vi "Super Talon Test 2016.vi"() -> ()   [LabVIEW 2015]
doc: "This example shows how to control motor speed using CAN Jaguar and a quadrature encoder. For details setting up and understanding CAN Jaguar, see the Can Jaguar Fundamentals tutorial accessable from the LabVIEW Getting Started Window.\n\nTo control the motor speed, a PID control loop runs on the Jaguar. Notice that the encoder is wired directly to the Jaguar. One advantage of this is that the PID control does not use resources on the roboRIO. One disadvantage is that the PID code cannot be viewed or changed. However, the control can be tuned by changing the PID Parameters.\n\nOn the diagram, notice that the PID tuning parameters are only applied once before the motor is enabled. To learn about changing PID parameters while the program is running, see the CAN Position Control Encoder example. Since the control loop runs on the Jaguar, the LabVIEW loop delay is set to a slow 100ms. In fact the only reason this loop needs to run is to send a new set speed and read the actual speed.\n\nCorrect tuning parameters for a PID controller are dependent on the complete system of the motor and the load. It will be difficult to tune this system if there is no load attached to the motor. While this example is not a PID tutorial, the following information may help in understanding how to tune your PID control system.\n\nP (proportional) depends on the present error, I (integral) on the accumulation of past errors, and D (derivative) is a prediction of future errors, based on the current rate of change. The proportional parameter (P) will reduce the rise time and will reduce, but never eliminate, the steady-state error. The integral parameter (I) will eliminate the steady-state error, but may make the transient response worse. The derivative parameter (D) will increase the stability of the system, reducing the overshoot, and improving the transient response. The effects of each parameter are summarized in a table on the front panel.\n\nThis example expects a USB cable connected from your development PC to the Type B USB Jack (next to the power input) on the roboRIO.\n\nThis example requires the Driver Station to be running with Teleoperated Enabled."
uses:
  <vilib>/Rock Robotics/WPI/CAN/TalonSRX/WPI_CANTalonSRX_APIControlMode.ctl
  <vilib>/Rock Robotics/WPI/CAN/TalonSRX/WPI_CANTalonSRX_APIFeedbackSelect.ctl
  <vilib>/Rock Robotics/WPI/MotorControl/WPI_MotorControlOpenCANTalonSRX.vi
panel:
  in  "Stop All":bool
  in  "Start All":bool
  in  "Tab Control 2":T1(tab)
  out "Actual Speed (RPM)":dbl
  in  "P":dbl=1.0
  in  "D":dbl
  in  "F":dbl=0.01
  in  "I":dbl
  in  "Target Value":dbl
  out "Actual Position (Rotations)":dbl
  out "Percent VBus":dbl
  out "A/D Value":dbl
  out "Test Running":string
  in  "Control Mode":string(combo)
  in  "Motor Address":u64
  in  "Tab Control":T2(tab)
  out "Voltage Feedback Chart":cluster{dbl, dbl}(graph)
  out "Speed Feedback Chart":cluster{dbl, dbl}(graph)
  out "Position Feedback Chart":cluster{dbl, dbl}(graph)
  out "Potentiometer Position Feedback":cluster{dbl, dbl}(graph)
  in  "Stop Motor 1":bool
  in  "Forward Limit Switch":bool
  in  "Reverse Limit Switch":bool
  in  "Switches Normally Open":bool
  in  "Start Motor 1":bool
  in  "I Zone":dbl=0.01
  in  "I Zone 2":dbl=0.01
  in  "Start Motor 2":bool
  in  "Motor Address 2":u64
  in  "Control Mode 2":string(combo)
  in  "Target Value 2":dbl
  in  "I 2":dbl
  in  "F 2":dbl=0.01
  in  "D 2":dbl caption="D"
  in  "P 2":dbl=1.0 caption="P"
  out "Test Running 2":string
  out "Percent VBus 2":dbl
  out "A/D Value 2":dbl
  out "Actual Speed (RPM) 2":dbl
  out "Actual Position (Rotations) 2":dbl
  in  "Switches Normally Open 2":bool
  in  "Reverse Limit Switch 2":bool
  in  "Forward Limit Switch 2":bool
  in  "Tab Control 3":T2(tab)
  out "Voltage Feedback Chart 2":cluster{dbl, dbl}(graph)
  out "Speed Feedback Chart 2":cluster{dbl, dbl}(graph)
  out "Position Feedback Chart 2":cluster{dbl, dbl}(graph)
  out "Potentiometer Position Feedback 2":cluster{dbl, dbl}(graph)
  in  "Stop Motor 2":bool
  in  "I Zone 3":dbl=0.01
  in  "Start Motor 3":bool
  in  "Motor Address 3":u64
  in  "Control Mode 3":string(combo)
  in  "Target Value 3":dbl
  in  "I 3":dbl
  in  "F 3":dbl=0.01
  in  "D 3":dbl caption="D"
  in  "P 3":dbl=1.0 caption="P"
  out "Test Running 3":string
  out "Percent VBus 3":dbl
  out "A/D Value 3":dbl
  out "Actual Speed (RPM) 3":dbl
  out "Actual Position (Rotations) 3":dbl
  in  "Switches Normally Open 3":bool
  in  "Reverse Limit Switch 3":bool
  in  "Forward Limit Switch 3":bool
  in  "Tab Control 4":T2(tab)
  out "Voltage Feedback Chart 3":cluster{dbl, dbl}(graph)
  out "Speed Feedback Chart 3":cluster{dbl, dbl}(graph)
  out "Position Feedback Chart 3":cluster{dbl, dbl}(graph)
  out "Potentiometer Position Feedback 3":cluster{dbl, dbl}(graph)
  in  "Stop Motor 3":bool
  in  "I Zone 4":dbl=0.01
  in  "Start Motor 4":bool
  in  "Motor Address 4":u64
  in  "Control Mode 4":string(combo)
  in  "Target Value 4":dbl
  in  "I 4":dbl
  in  "F 4":dbl=0.01
  in  "D 4":dbl caption="D"
  in  "P 4":dbl=1.0 caption="P"
  out "Test Running 4":string
  out "Percent VBus 4":dbl
  out "A/D Value 4":dbl
  out "Actual Speed (RPM) 4":dbl
  out "Actual Position (Rotations) 4":dbl
  in  "Switches Normally Open 4":bool
  in  "Reverse Limit Switch 4":bool
  in  "Forward Limit Switch 4":bool
  in  "Stop Motor 4":bool
  in  "Tab Control 5":T2(tab)
  out "Voltage Feedback Chart 4":cluster{dbl, dbl}(graph)
  out "Speed Feedback Chart 4":cluster{dbl, dbl}(graph)
  out "Position Feedback Chart 4":cluster{dbl, dbl}(graph)
  out "Potentiometer Position Feedback 4":cluster{dbl, dbl}(graph)
  out "Error Out":errorcluster
  in  "Error In":errorcluster
  # "Set these inputs before running."
  # "Tuning parameters"
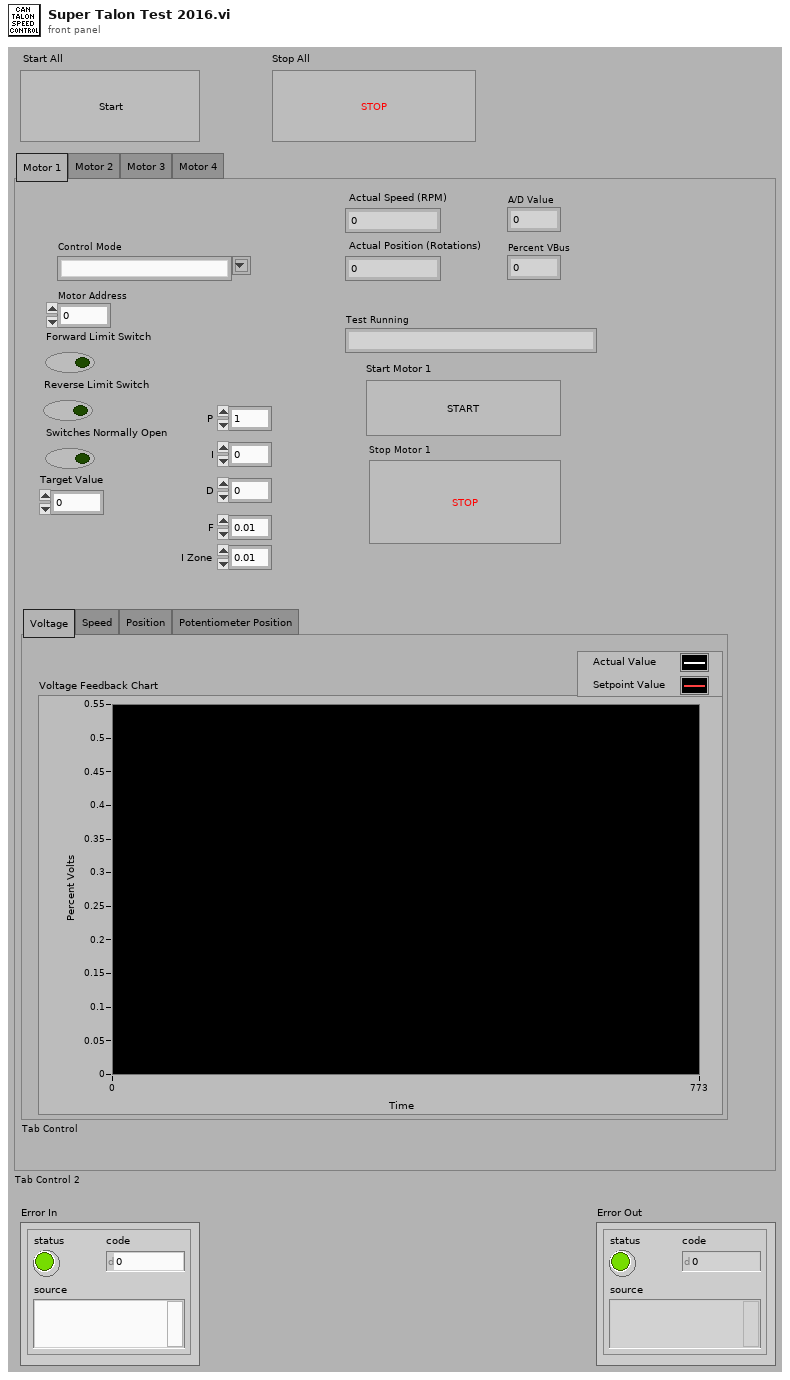
[diagram p1: front panel]
types:
  T1 = enum32{"Motor 1", "Motor 2", "Motor 3", "Motor 4"}
  T2 = enum32{"Voltage", "Speed", "Position", "Potentiometer Position"}
  T3 = typedef "WPI_CANTalonSRX_APIFeedbackSelect.ctl" = enum16{"Digital Quadrature Encoder", "Analog Potentiometer", "Analog Encoder", "Count on Quad-A (Rising-Edge)", "Count on Quad-A (Falling-Edge)", "CTR Magnetic Enc (Absolute)", "CTR Magnetic Enc (Relative)", "Pulse Width"}
  T4 = typedef "WPI_CANTalonSRX_APIControlMode.ctl" = enum8{"Percent VBus", "Speed", "Position", "Slave", "Unchanged / Invalid", "Voltage Compensation", "Current", "Motion Profile"}
  T5 = typedef "WPI_MotorControlDeviceRef.ctl" = cluster{"DeviceStatus":errorcluster, "Type":T6, "PWM":cluster{"PWM Channel":T7, "DeadBand":T8}, "CAN":cluster{"Device Number":u8, "Control Mode":T9, "Semaphore":T10, "Max Vout":dbl, "TalonSRX Control Mode":T4}, "Invert":bool}
  T6 = typedef "WPI_MotorControlType.ctl" = enum16{"PWM", "CAN", "CANTalonSRX"}
  T7 = typedef "FPGA_DIOPWMChannel.ctl" = enum8{"PWM 0", "PWM 1", "PWM 2", "PWM 3", "PWM 4", "PWM 5", "PWM 6", "PWM 7", "PWM 8", "PWM 9", "PWM MXP 0", "PWM MXP 1", "PWM MXP 2", "PWM MXP 3", "PWM MXP 4", "PWM MXP 5", "PWM MXP 6", "PWM MXP 7", "PWM MXP 8", "PWM MXP 9", "Invalid"}
  T8 = typedef "WPI_PWMDeadband.ctl" = cluster{"Name":string, "maxPositivePwm":i32, "minPositivePwm":i32, "centerPwm":i32, "maxNegativePwm":i32, "minNegativePwm":i32, "angularRange":u16}
  T9 = typedef "WPI_CANJaguar_ControlMode.ctl" = enum8{"Percent VBus", "Current", "Speed", "Position", "Voltage"}
  T10 = typedef "Semaphore RefNum" = refnum<k1>
  T11 = typedef "WPI_CANTalonSRX_GlobalStatus.ctl" = cluster{"Applied Throttle":dbl, "Module Enabled":bool, "CAN Error":errorcluster, "Closed Loop Error":dbl, "Forward Limit Switch Closed":bool, "Reverse Limit Switch Closed":bool, "Sensor Position":dbl, "Sensor Velocity":dbl, "Current":dbl, "Sticky Fault - Over Temp":bool, "Sticky Fault - Under Voltage":bool, "Sticky Fault - Forward Limit":bool, "Sticky Fault - Reverse Limit":bool, "Sticky Fault - Forward Soft Limit":bool, "Sticky Fault - Reverse Soft Limit":bool, "Brake is Enabled":bool, "Encoder Position":dbl, "Encoder Velocity":dbl, "Encoder Index Count":dbl, "Encoder A Pin State":bool, "Encoder B Pin State":bool, "Encoder Index Pin State":bool, "Analog In":dbl, "Analog In Velocity":dbl, "Temperature (C)":dbl, "Battery Voltage":dbl, "Control 5 Is Supported":bool, "Current Profile Slot Select":dbl, "Pos Div 8":bool, "Vel Div 4":bool, "Pulse Width Position":i32, "Pulse Width Velocity":i32, "Pulse Width Rise To Rise (us)":i32, "Pulse Width Rise To Fall (us)":i32, "Mot Prof Active Is Under Run":bool, "Mot Prof Active Has Under Run":bool, "Mot Prof Active Is Last":bool, "Mot Prof Active Velocity Only":bool, "Mot Prof Active Is Valid":bool, "Mot Prof Buffer Is Full":bool, "Mot Prof Active Profile Slot Select":i32, "Mot Prof NextID":i32, "Mot Prof Count":i32, "Mot Prof Active Velocity":dbl, "Mot Prof Active Position":dbl, "Mot Prof Output Enable":i32}
  T12 = cluster{"Applied Throttle":dbl, "Target Value 2":dbl}
  T13 = cluster{"Applied Throttle":dbl, "Target Value":dbl}
  T14 = cluster{"Applied Throttle":dbl, "Target Value 3":dbl}
  T15 = cluster{"Applied Throttle":dbl, "Target Value 4":dbl}
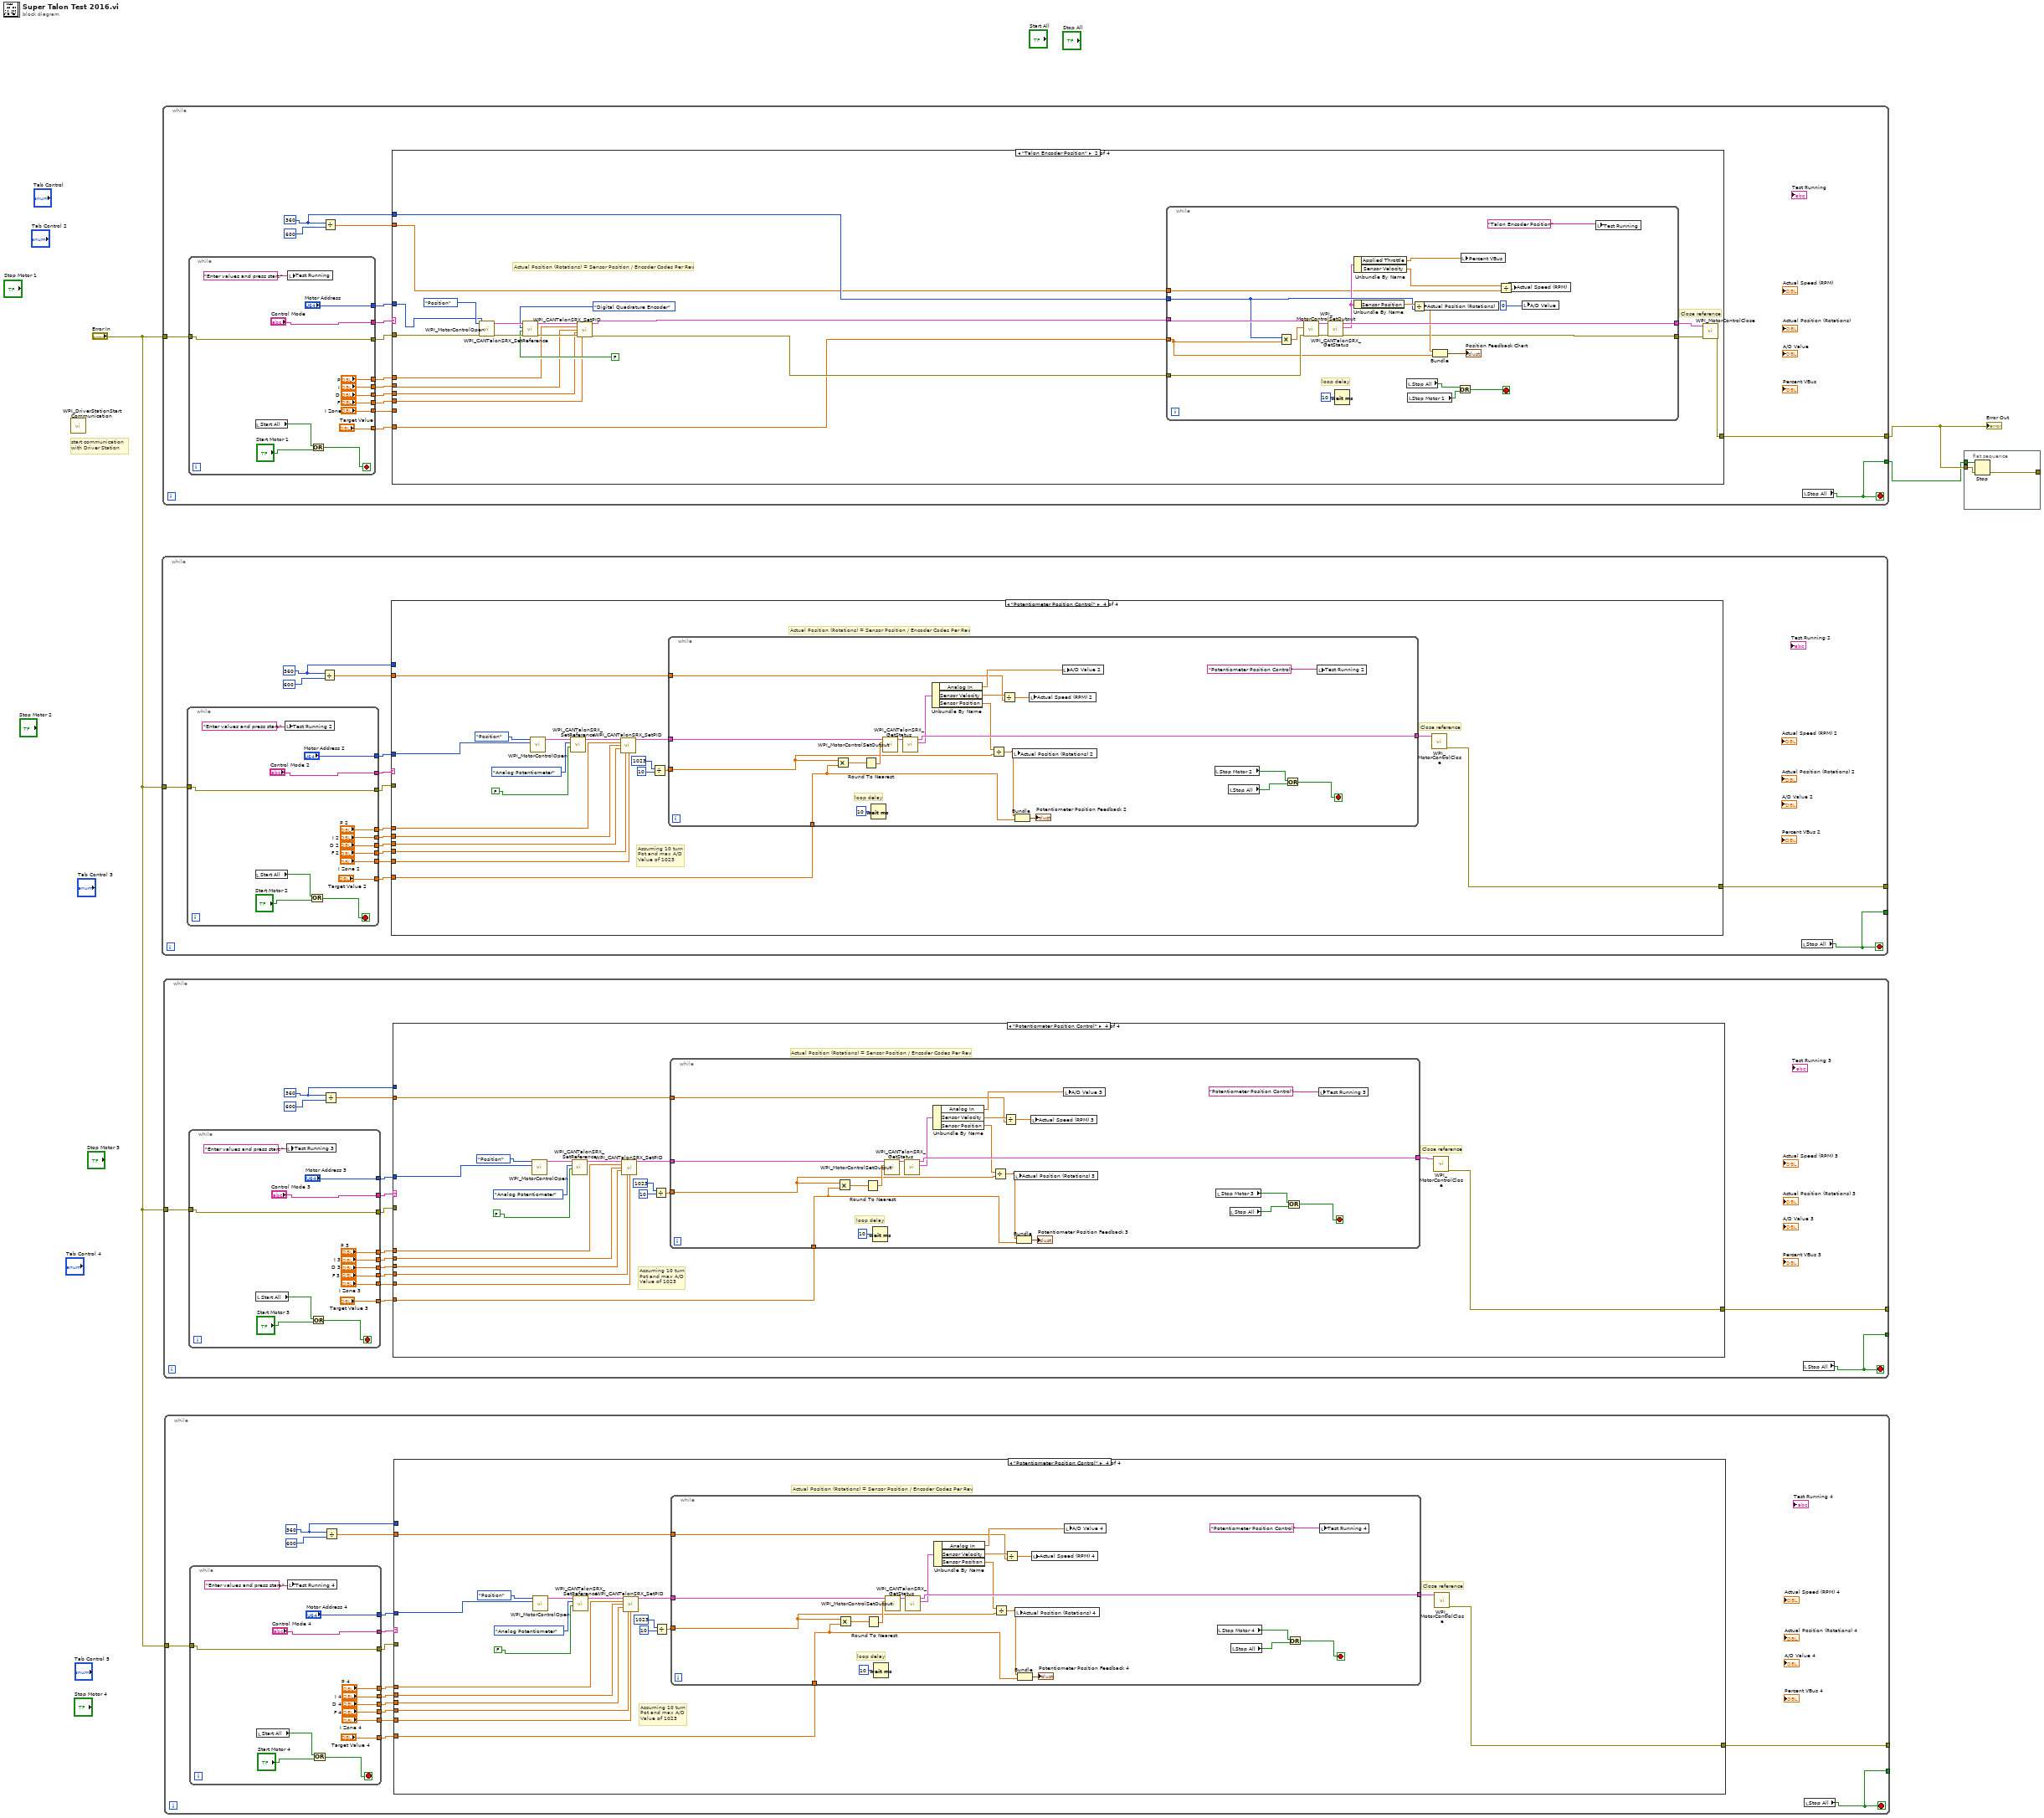
[diagram p0: block diagram]
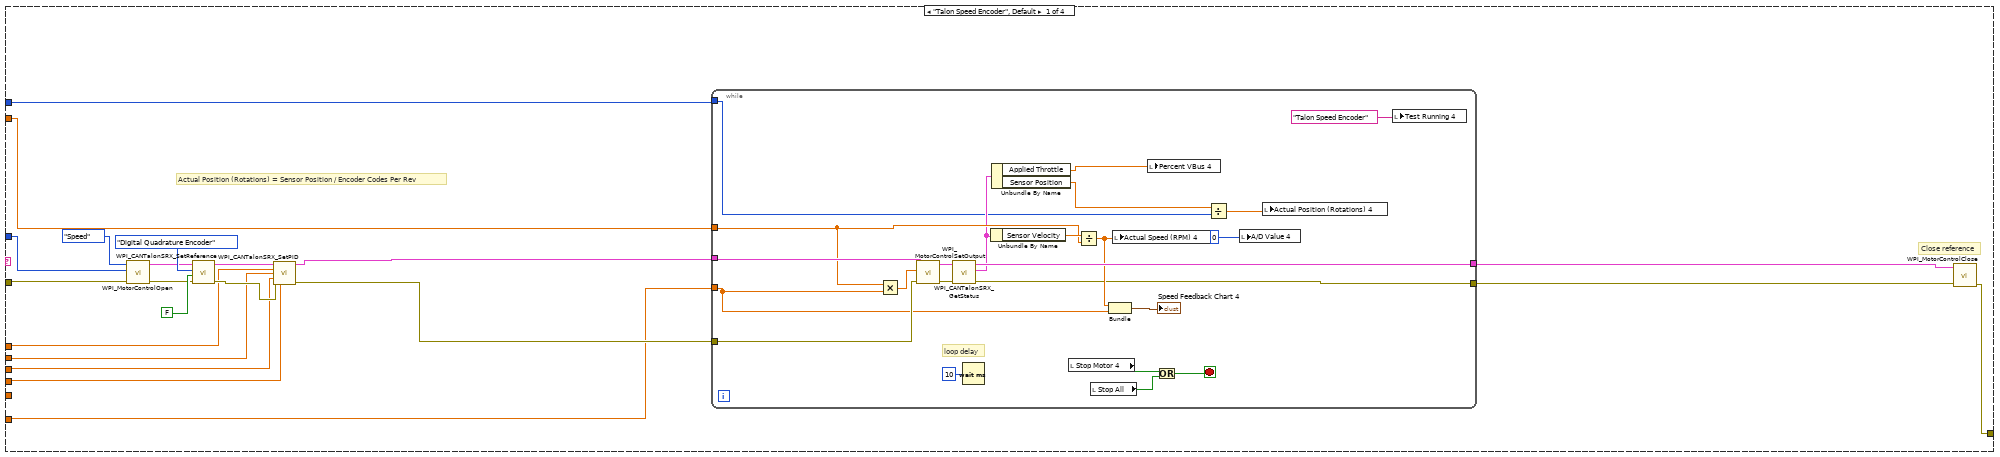
[diagram p2: hidden frame]
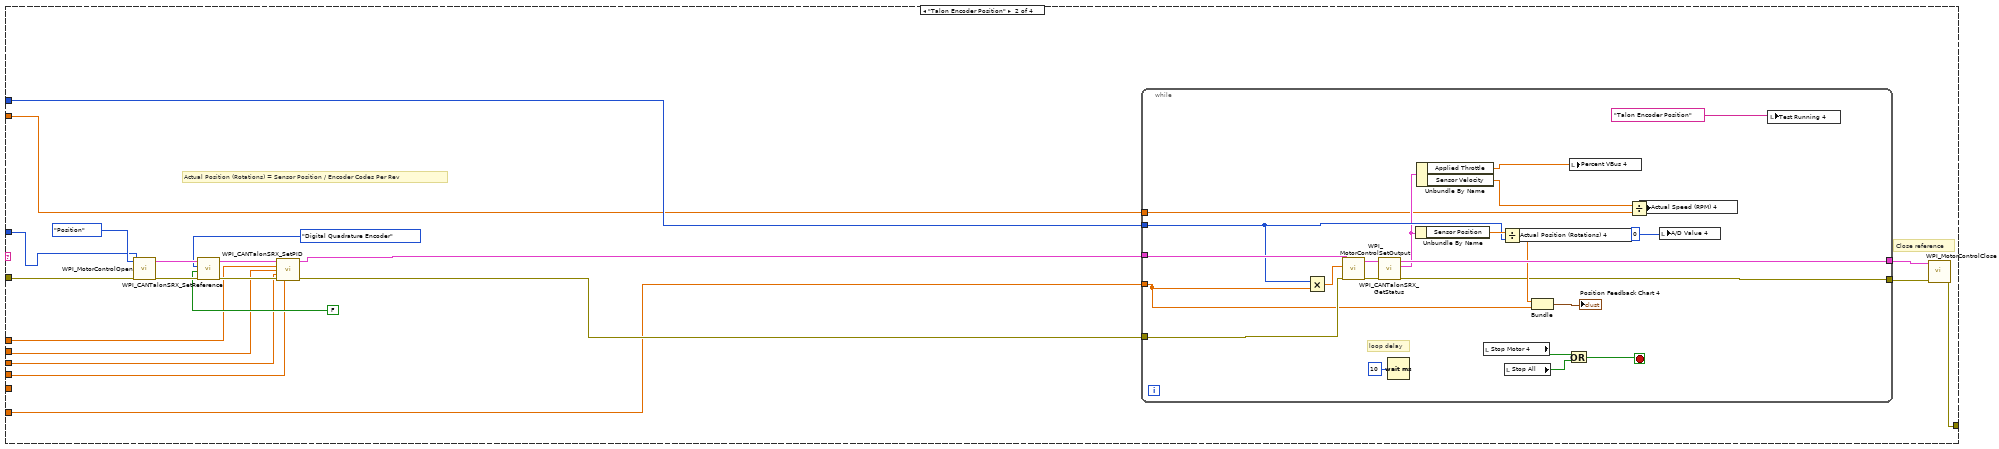
[diagram p3: hidden frame]
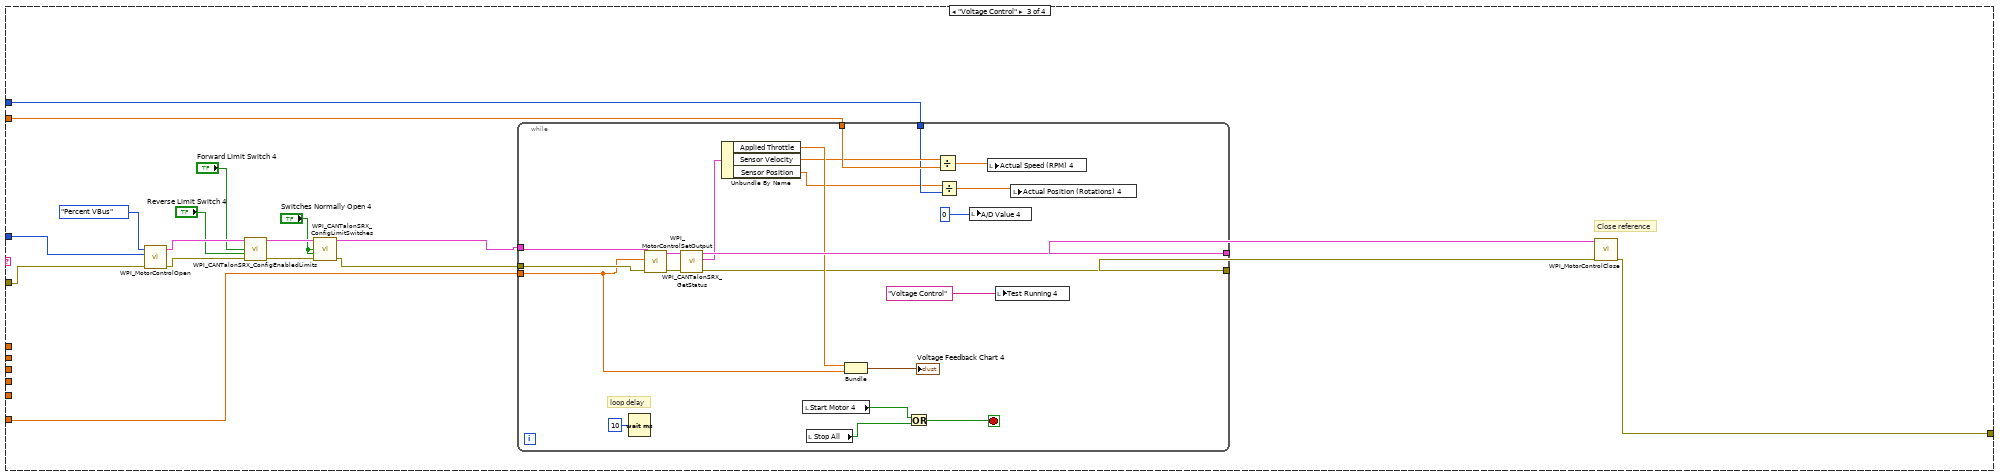
[diagram p4: hidden frame]
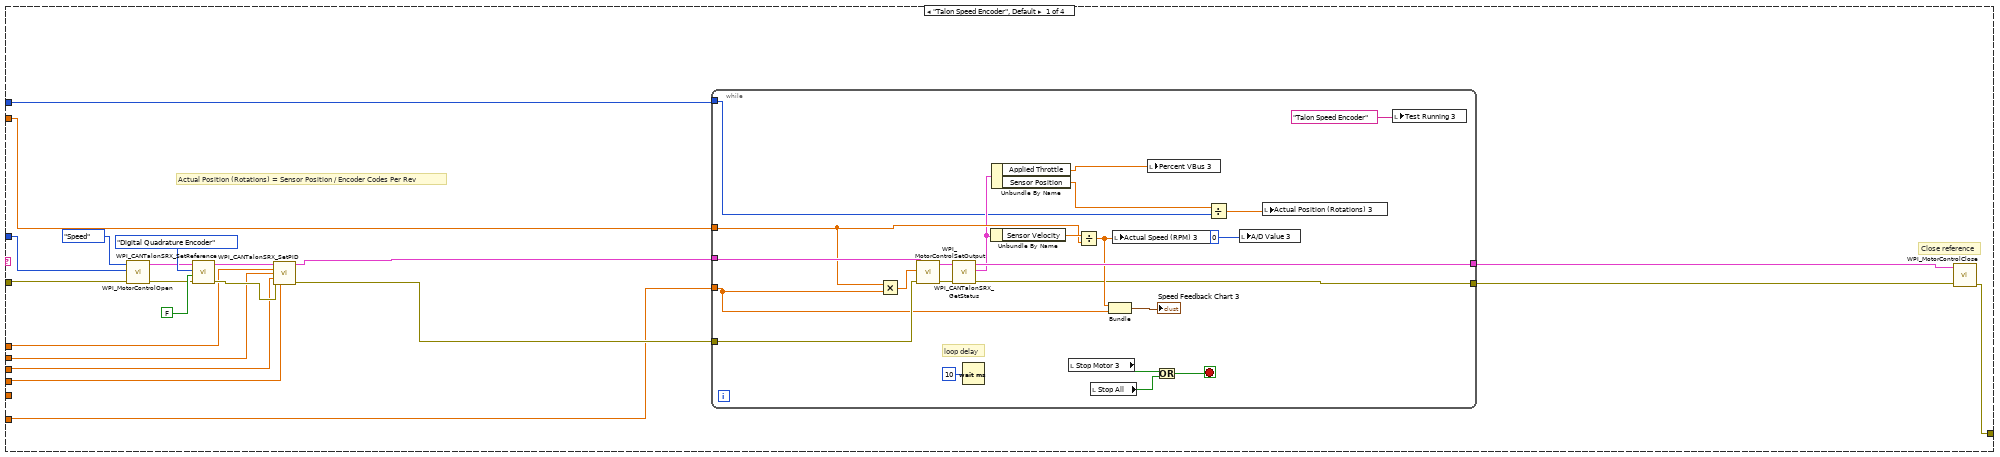
[diagram p5: hidden frame]
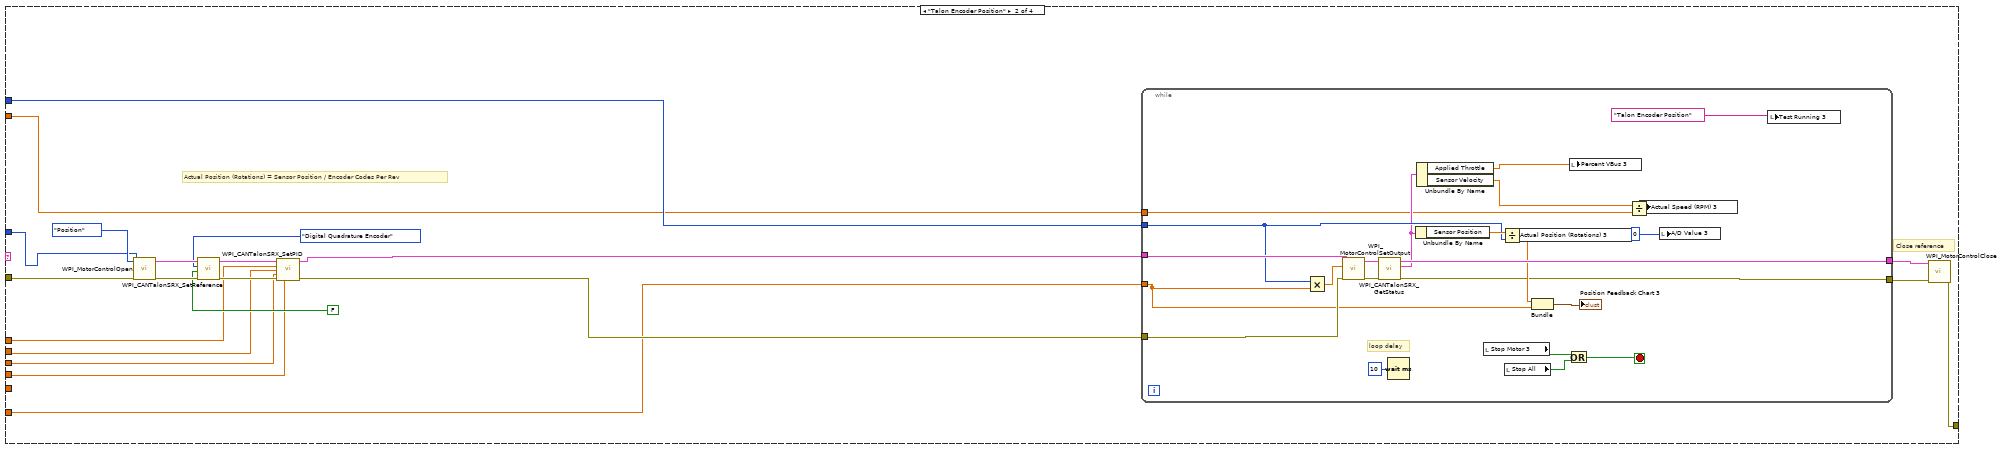
[diagram p6: hidden frame]
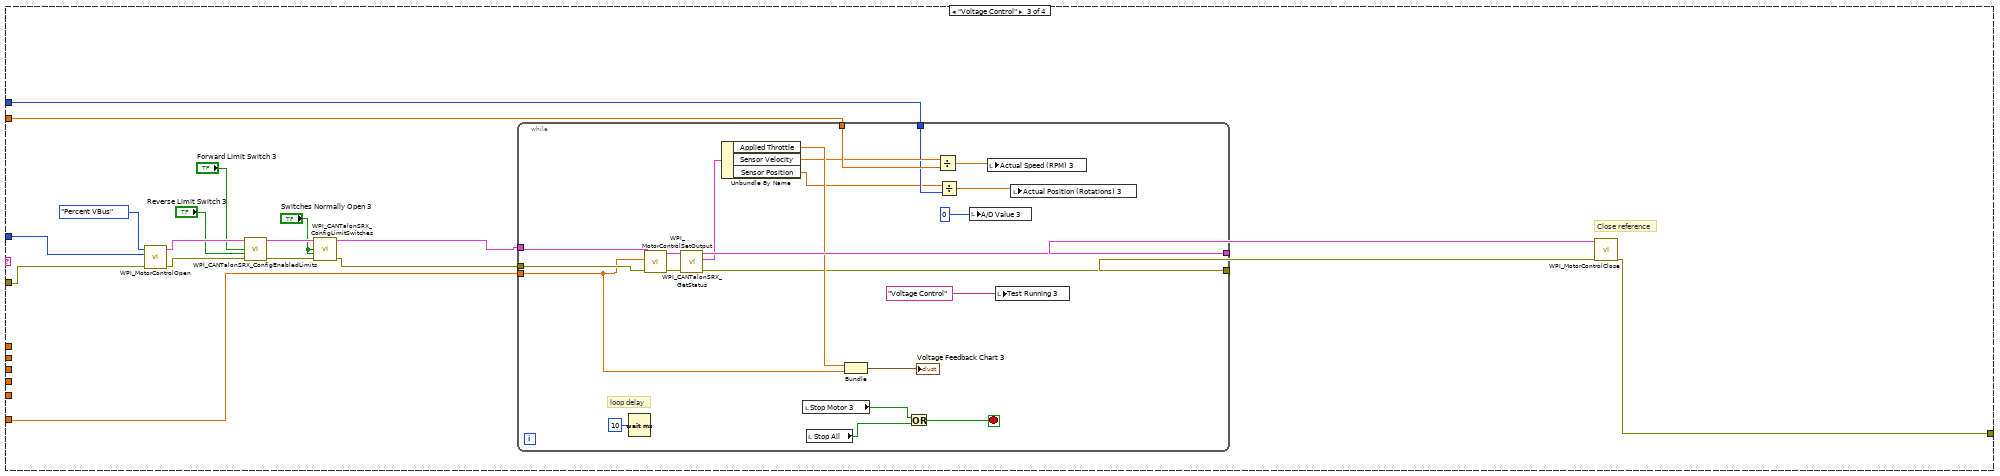
[diagram p7: hidden frame]
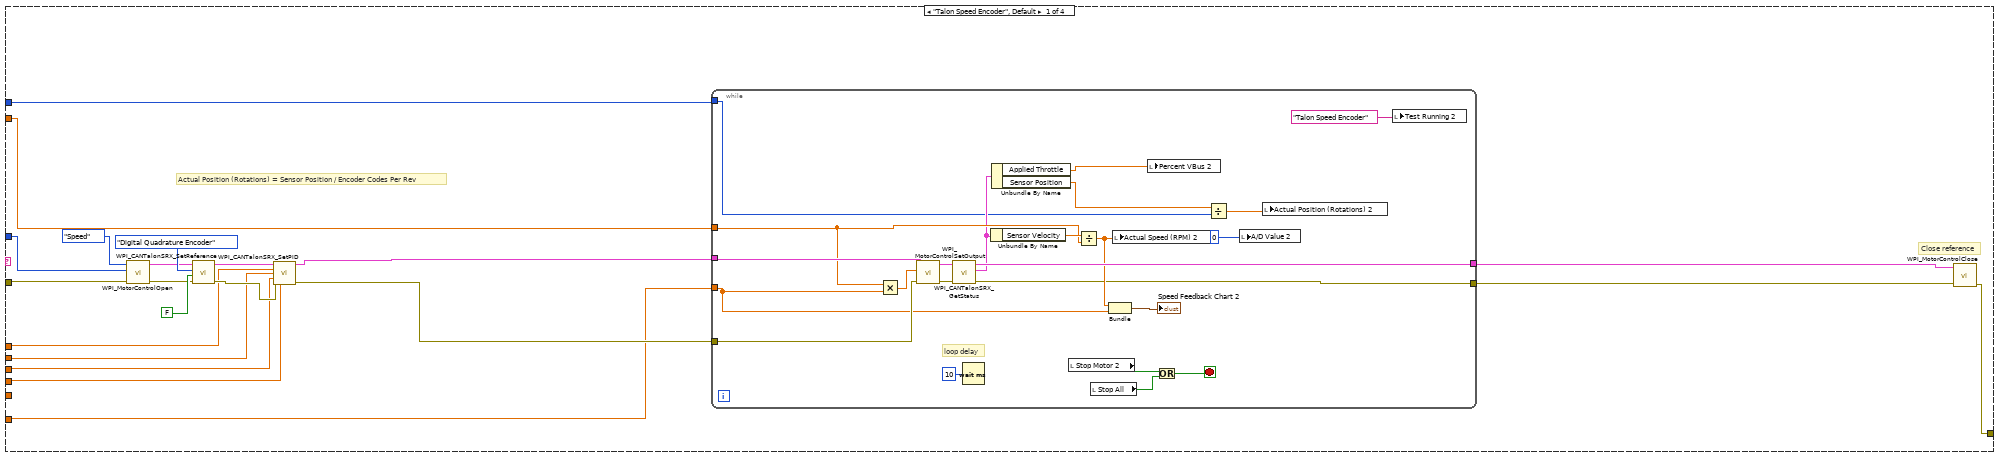
[diagram p8: hidden frame]
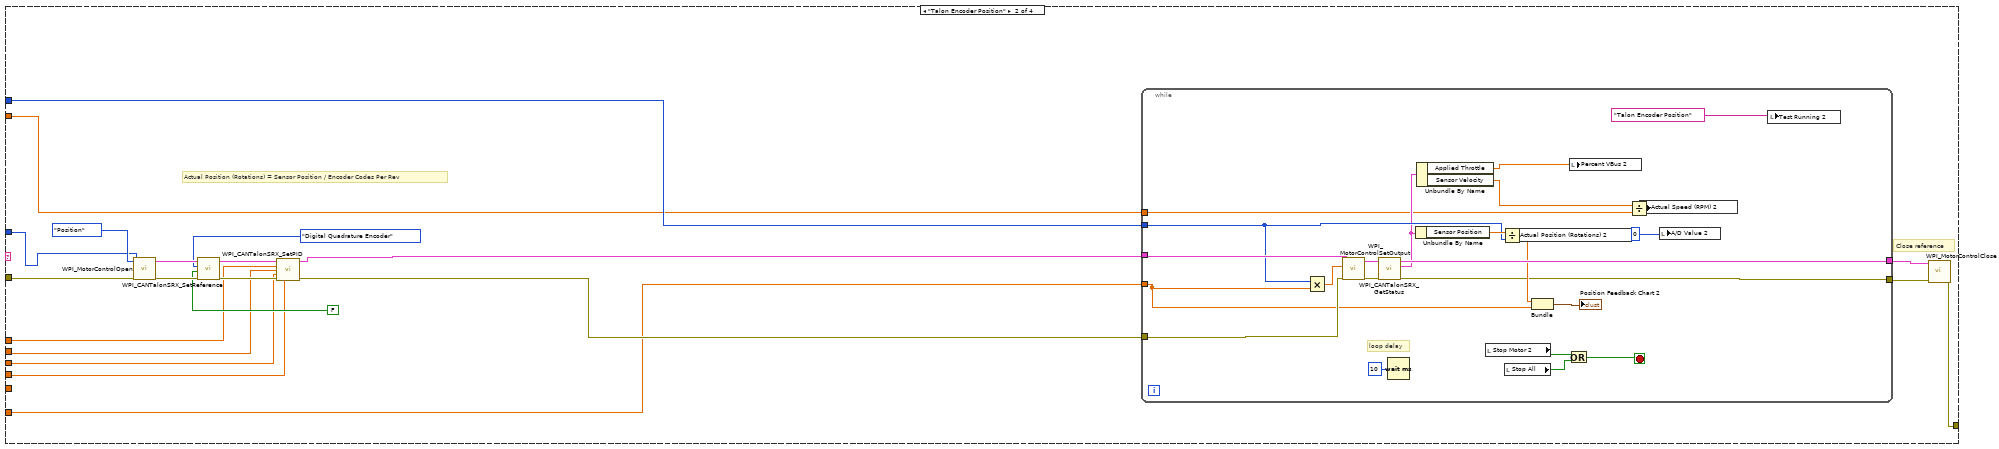
[diagram p9: hidden frame]
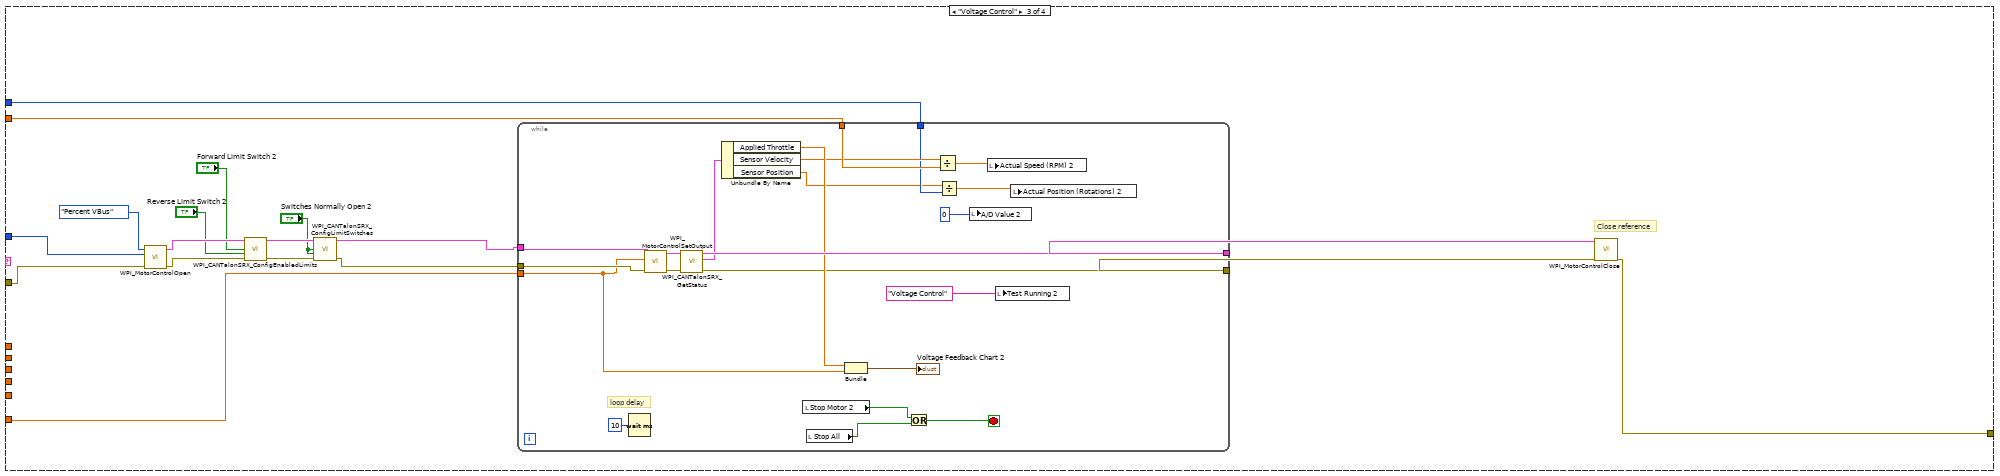
[diagram p10: hidden frame]
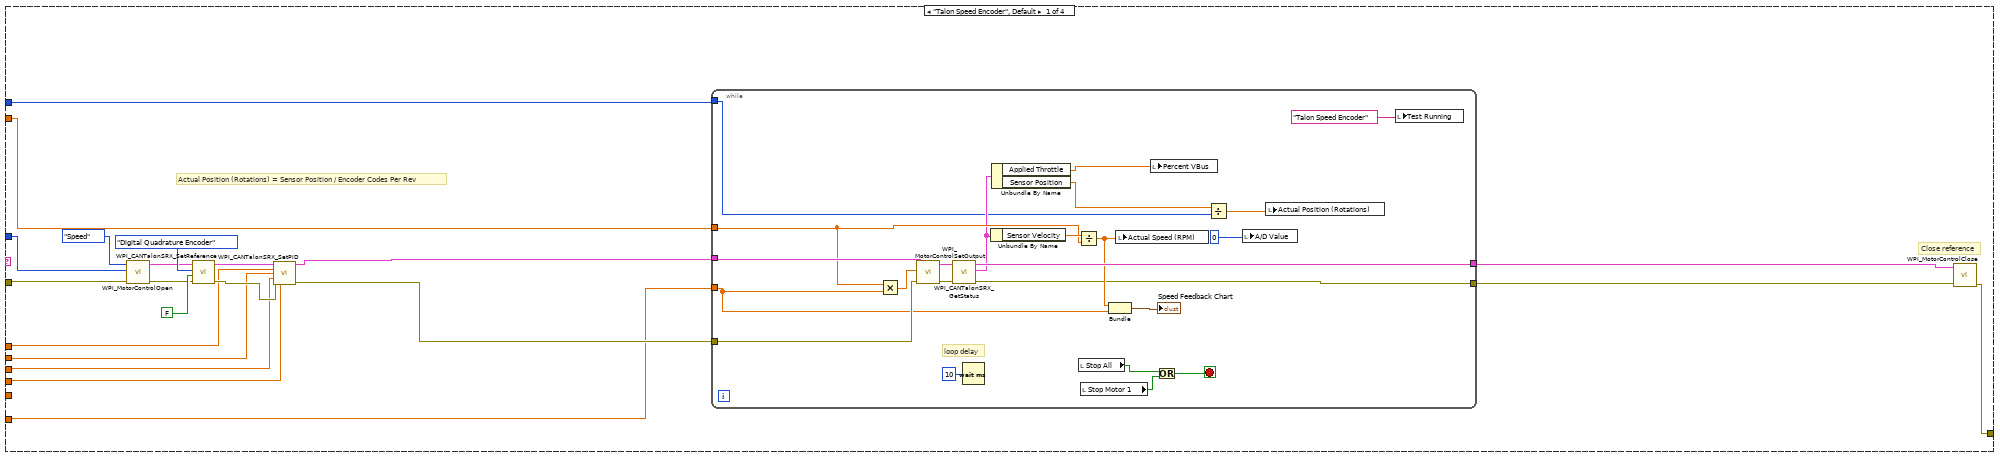
[diagram p11: hidden frame]
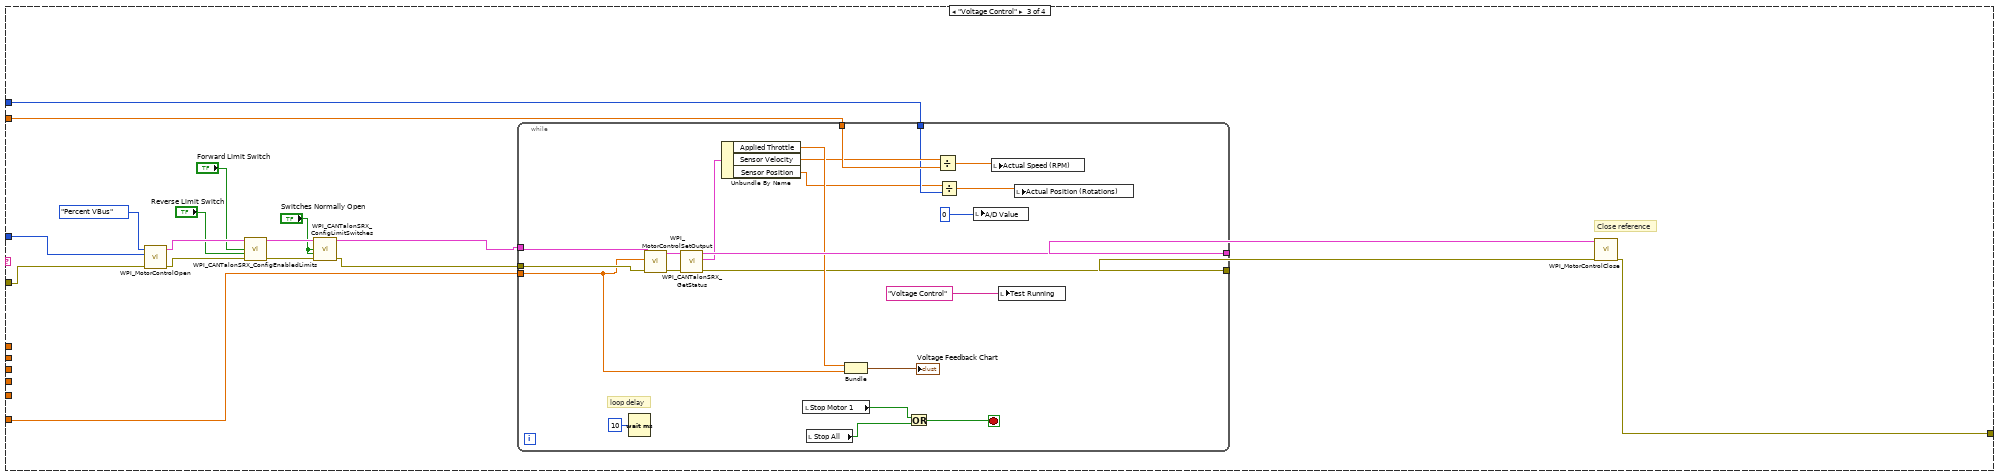
[diagram p12: hidden frame]
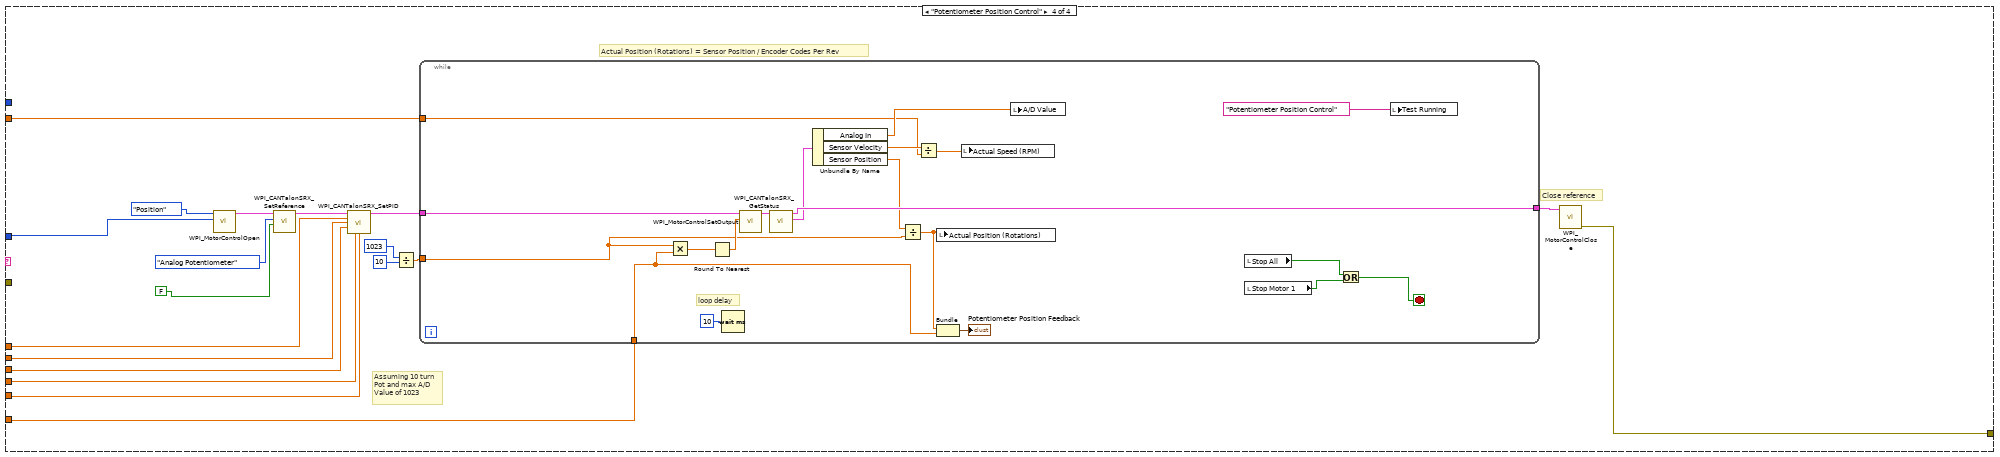
[diagram p13: hidden frame]
diagram:
  # "start communication with Driver Station"
  n1 = call <vilib>:"WPI_DriverStationStart Communication.vi"() -> ()  [unwired: 2 in, 10 out]
  n2 = while {
    tunnel: "Error In" -> [w7]
    tunnel: [w6] -> _
    tunnel: [w4] -> _
    stop <- w4 stop-if-true
    w16 = 360
    n3 = while {
      tunnel: ["P 2"] -> w15
      tunnel: ["I 2"] -> w14
      tunnel: ["D 2"] -> w13
      tunnel: ["F 2"] -> w12
      tunnel: ["Target Value 2"] -> w11
      tunnel: ["Control Mode 2"] -> w10
      tunnel: ["Motor Address 2"] -> w9
      tunnel: [w24] -> w8
      tunnel: w7 -> [w24]
      tunnel: ["I Zone 2"] -> w5
      stop <- w20 stop-if-true
      n4 = local read "Start All"() -> (w22:bool)
      n5 = local write "Test Running 2"("Enter values and press start.") -> ()
      n6 = Or(x=w22, y="Start Motor 2") -> (x .or. y?=w20:bool)
    }
    n7 = Divide(x=w16, y=600) -> (x/y=w17:dbl)
    n8 = case shown="\"Potentiometer Position Control\"" w10 {
      tunnel: w17 -> [w41 w76 w133 w162]
      tunnel: w16 -> [w42 w77 w134 _]
      tunnel: w8 -> [w40 w84 w131 _]
      tunnel: [w34 w78 w129 w163] -> w6
      tunnel: w15 -> [w39 w83 _ w167]
      tunnel: w14 -> [w38 w82 _ w166]
      tunnel: w13 -> [w37 w81 _ w161]
      tunnel: w12 -> [w36 w80 _ w165]
      tunnel: w11 -> [w35 w79 w130 w164]
      tunnel: w9 -> [w32 w85 w132 w168]
      tunnel: w5 -> [_ _ _ w160]
      frame "Talon Speed Encoder", Default {
        # "Actual Position (Rotations) = Sensor Position / Encoder Codes Per Rev"
        # "Close reference"
        n9 = call-poly <vilib>:"WPI_MotorControlOpen.vi"("error in (no error)"=w40, "Device Number"=w32, "Control Mode"=WPI_CANTalonSRX_APIControlMode."Speed") -> ("error out"=w46:errorcluster, "MotorControlDeviceRef"=w49:T5)  [unwired: 2 in, 5 out]
        n10 = call <vilib>:"WPI_CANTalonSRX_SetReference.vi"("error in (no error)"=w46, "Reverse Feedback Sensor"=FALSE, "Feedback Reference"=WPI_CANTalonSRX_APIFeedbackSelect."Digital Quadrature Encoder", "CAN Talon SRX Ref"=w49) -> ("error out"=w45:errorcluster, "CAN Talon SRX Ref"=w48:T5)  [unwired: 6 in]
        n11 = call <vilib>:"WPI_CANTalonSRX_SetPID.vi"("CAN Talon SRX Ref"=w48, "P"=w39, "I"=w38, "D"=w37, "error in (no error)"=w45, "F"=w36) -> ("CAN Talon SRX Ref"=w47:T5, "error out"=w44:errorcluster)  [unwired: 8 in]
        n12 = while {
          tunnel: w47 -> [w69]
          tunnel: [w74] -> w52
          tunnel: w41 -> [w68]
          tunnel: w42 -> [w62]
          tunnel: w44 -> [w60]
          tunnel: [w58] -> w43
          tunnel: w35 -> [w57]
          stop <- w53 stop-if-true
          # "loop delay"
          n13 = Multiply(x=w68, y=w57) -> (x*y=w71:dbl)
          n14 = call <vilib>:"WPI_MotorControlSetOutput.vi"("error in (no error)"=w60, "Output"=w71, "MotorControlDevRef"=w69) -> ("error out"=w59:errorcluster, "MotorControlDevRef"=w73:T5)  [unwired: 6 in, 1 out]
          n15 = call <vilib>:"WPI_CANTalonSRX_GetStatus.vi"("error in (no error)"=w59, "CAN Talon SRX Ref"=w73) -> ("error out"=w58:errorcluster, "Talon SRX Status"=w64:T11, "CAN Talon SRX Ref"=w74:T5)  [unwired: 7 in]
          n16 = Wait (ms)(milliseconds to wait=u32 10) -> ()  [unwired: 1 out]
          n17 = Unbundle By Name(w64) -> ("Sensor Velocity"=w72:dbl)
          n18 = Unbundle By Name(w64) -> ("Applied Throttle"=w63:dbl, "Sensor Position"=w61:dbl)
          n19 = local read "Stop Motor 2"() -> (w54:bool)
          n20 = Divide(x=w72, y=w68) -> (x/y=w67:dbl)
          n21 = local read "Stop All"() -> (w55:bool)
          n22 = Bundle(w67, "Target Value 2"=w57) -> (→"Speed Feedback Chart 2":cluster{dbl, "Target Value 2":dbl})  [unwired: 1 in]
          n23 = local write "Actual Speed (RPM) 2"(w67) -> ()
          n24 = local write "Percent VBus 2"(w63) -> ()
          n25 = Or(x=w54, y=w55) -> (x .or. y?=w53:bool)
          n26 = Divide(x=w61, y=w62) -> (x/y=w66:dbl)
          n27 = local write "A/D Value 2"(0) -> ()
          n28 = local write "Actual Position (Rotations) 2"(w66) -> ()
          n29 = local write "Test Running 2"("Talon Speed Encoder") -> ()
        }
        n30 = call <vilib>:"WPI_MotorControlClose.vi"("error in (no error)"=w43, "MotorControlDevRef"=w52) -> ("error out"=w34:errorcluster)  [unwired: 9 in]
      }
      frame "Talon Encoder Position" {
        # "Actual Position (Rotations) = Sensor Position / Encoder Codes Per Rev"
        # "Close reference"
        n31 = call-poly <vilib>:"WPI_MotorControlOpen.vi"("error in (no error)"=w84, "Device Number"=w85, "Control Mode"=WPI_CANTalonSRX_APIControlMode."Position") -> ("error out"=w93:errorcluster, "MotorControlDeviceRef"=w90:T5)  [unwired: 2 in, 5 out]
        n32 = call <vilib>:"WPI_CANTalonSRX_SetReference.vi"("error in (no error)"=w93, "Reverse Feedback Sensor"=FALSE, "Feedback Reference"=WPI_CANTalonSRX_APIFeedbackSelect."Digital Quadrature Encoder", "CAN Talon SRX Ref"=w90) -> ("error out"=w94:errorcluster, "CAN Talon SRX Ref"=w91:T5)  [unwired: 6 in]
        n33 = call <vilib>:"WPI_CANTalonSRX_SetPID.vi"("CAN Talon SRX Ref"=w91, "P"=w83, "I"=w82, "D"=w81, "error in (no error)"=w94, "F"=w80) -> ("CAN Talon SRX Ref"=w92:T5, "error out"=w95:errorcluster)  [unwired: 8 in]
        n34 = while {
          tunnel: w92 -> [w113]
          tunnel: [w118] -> w86
          tunnel: w77 -> [w112]
          tunnel: w95 -> [w106]
          tunnel: [w104] -> w96
          tunnel: w79 -> [w103]
          tunnel: w76 -> [w102]
          stop <- w97 stop-if-true
          # "loop delay"
          n35 = Multiply(x=w112, y=w103) -> (x*y=w115:dbl)
          n36 = call <vilib>:"WPI_MotorControlSetOutput.vi"("error in (no error)"=w106, "Output"=w115, "MotorControlDevRef"=w113) -> ("error out"=w105:errorcluster, "MotorControlDevRef"=w117:T5)  [unwired: 6 in, 1 out]
          n37 = call <vilib>:"WPI_CANTalonSRX_GetStatus.vi"("error in (no error)"=w105, "CAN Talon SRX Ref"=w117) -> ("error out"=w104:errorcluster, "Talon SRX Status"=w108:T11, "CAN Talon SRX Ref"=w118:T5)  [unwired: 7 in]
          n38 = Wait (ms)(milliseconds to wait=u32 10) -> ()  [unwired: 1 out]
          n39 = Unbundle By Name(w108) -> ("Sensor Position"=w116:dbl)
          n40 = Unbundle By Name(w108) -> ("Applied Throttle"=w101:dbl, "Sensor Velocity"=w107:dbl)
          n41 = local read "Stop Motor 2"() -> (w99:bool)
          n42 = Divide(x=w116, y=w112) -> (x/y=w111:dbl)
          n43 = local read "Stop All"() -> (w98:bool)
          n44 = local write "Actual Position (Rotations) 2"(w111) -> ()
          n45 = Bundle(w111, "Target Value 2"=w103) -> (→"Position Feedback Chart 2":cluster{dbl, "Target Value 2":dbl})  [unwired: 1 in]
          n46 = Or(x=w99, y=w98) -> (x .or. y?=w97:bool)
          n47 = local write "Percent VBus 2"(w101) -> ()
          n48 = Divide(x=w107, y=w102) -> (x/y=w110:dbl)
          n49 = local write "Actual Speed (RPM) 2"(w110) -> ()
          n50 = local write "A/D Value 2"(0) -> ()
          n51 = local write "Test Running 2"("Talon Encoder Position") -> ()
        }
        n52 = call <vilib>:"WPI_MotorControlClose.vi"("error in (no error)"=w96, "MotorControlDevRef"=w86) -> ("error out"=w78:errorcluster)  [unwired: 9 in]
      }
      frame "Voltage Control" {
        # "Close reference"
        n53 = call-poly <vilib>:"WPI_MotorControlOpen.vi"("error in (no error)"=w131, "Device Number"=w132, "Control Mode"=WPI_CANTalonSRX_APIControlMode."Percent VBus") -> ("error out"=w125:errorcluster, "MotorControlDeviceRef"=w128:T5)  [unwired: 2 in, 5 out]
        n54 = call <vilib>:"WPI_CANTalonSRX_ConfigEnabledLimits.vi"("CAN Talon SRX Ref"=w128, "Forward Limit Switch Enable"="Forward Limit Switch 2", "Reverse Limit Switch Enable"="Reverse Limit Switch 2", "error in (no error)"=w125) -> ("CAN Talon SRX Ref"=w127:T5, "error out"=w124:errorcluster)  [unwired: 10 in]
        n55 = call <vilib>:"WPI_CANTalonSRX_ConfigLimitSwitches.vi"("CAN Talon SRX Ref"=w127, "Forward Limit Switch Normally Open"="Switches Normally Open 2", "Reverse Limit Switch Normally Open"="Switches Normally Open 2", "error in (no error)"=w124) -> ("CAN Talon SRX Ref"=w126:T5, "error out"=w123:errorcluster)  [unwired: 10 in]
        n56 = while {
          tunnel: w126 -> [w155]
          tunnel: [w158] -> w136
          tunnel: w133 -> [w154]
          tunnel: w134 -> [w150]
          tunnel: w123 -> [w146]
          tunnel: [w144] -> w135
          tunnel: w130 -> [w142]
          stop <- w138 stop-if-true
          # "loop delay"
          n57 = Wait (ms)(milliseconds to wait=u32 10) -> ()  [unwired: 1 out]
          n58 = call <vilib>:"WPI_MotorControlSetOutput.vi"("error in (no error)"=w146, "Output"=w142, "MotorControlDevRef"=w155) -> ("error out"=w145:errorcluster, "MotorControlDevRef"=w157:T5)  [unwired: 6 in, 1 out]
          n59 = call <vilib>:"WPI_CANTalonSRX_GetStatus.vi"("error in (no error)"=w145, "CAN Talon SRX Ref"=w157) -> ("error out"=w144:errorcluster, "Talon SRX Status"=w156:T11, "CAN Talon SRX Ref"=w158:T5)  [unwired: 7 in]
          n60 = Unbundle By Name(w156) -> ("Applied Throttle"=w153:dbl, "Sensor Velocity"=w151:dbl, "Sensor Position"=w149:dbl)
          n61 = local read "Stop Motor 2"() -> (w140:bool)
          n62 = local read "Stop All"() -> (w139:bool)
          n63 = Bundle("Applied Throttle"=w153, "Target Value 2"=w142) -> (→"Voltage Feedback Chart 2":T12)  [unwired: 1 in]
          n64 = Or(x=w140, y=w139) -> (x .or. y?=w138:bool)
          n65 = Divide(x=w151, y=w154) -> (x/y=w152:dbl)
          n66 = Divide(x=w149, y=w150) -> (x/y=w148:dbl)
          n67 = local write "A/D Value 2"(0) -> ()
          n68 = local write "Actual Speed (RPM) 2"(w152) -> ()
          n69 = local write "Test Running 2"("Voltage Control") -> ()
          n70 = local write "Actual Position (Rotations) 2"(w148) -> ()
        }
        n71 = call <vilib>:"WPI_MotorControlClose.vi"("error in (no error)"=w135, "MotorControlDevRef"=w136) -> ("error out"=w129:errorcluster)  [unwired: 9 in]
      }
      frame "Potentiometer Position Control" {
        # "Assuming 10 turn\nPot and max A/D\nValue of 1023"
        # "Actual Position (Rotations) = Sensor Position / Encoder Codes Per Rev"
        # "Close reference"
        n72 = call-poly <vilib>:"WPI_MotorControlOpen.vi"("Device Number"=w168, "Control Mode"=WPI_CANTalonSRX_APIControlMode."Position") -> ("MotorControlDeviceRef"=w175:T5)  [unwired: 3 in, 6 out]
        n73 = call <vilib>:"WPI_CANTalonSRX_SetReference.vi"("Reverse Feedback Sensor"=FALSE, "Feedback Reference"=WPI_CANTalonSRX_APIFeedbackSelect."Analog Potentiometer", "CAN Talon SRX Ref"=w175) -> ("CAN Talon SRX Ref"=w174:T5)  [unwired: 7 in, 1 out]
        n74 = call <vilib>:"WPI_CANTalonSRX_SetPID.vi"("CAN Talon SRX Ref"=w174, "P"=w167, "I"=w166, "D"=w161, "F"=w165, "I Zone"=w160) -> ("CAN Talon SRX Ref"=w171:T5)  [unwired: 8 in, 1 out]
        n75 = Divide(x=1023, y=10) -> (x/y=w172:dbl)
        n76 = while {
          tunnel: w171 -> [w192]
          tunnel: [w197] -> w178
          tunnel: w172 -> [w186]
          tunnel: w164 -> [w189]
          tunnel: w162 -> [w184]
          stop <- w179 stop-if-true
          # "loop delay"
          n77 = Multiply(x=w186, y=w189) -> (x*y=w191:dbl)
          n78 = Round To Nearest(number=w191) -> (nearest integer value=w190:dbl)
          n79 = Wait (ms)(milliseconds to wait=u32 10) -> ()  [unwired: 1 out]
          n80 = call <vilib>:"WPI_MotorControlSetOutput.vi"("Output"=w190, "MotorControlDevRef"=w192) -> ("MotorControlDevRef"=w196:T5)  [unwired: 7 in, 2 out]
          n81 = call <vilib>:"WPI_CANTalonSRX_GetStatus.vi"("CAN Talon SRX Ref"=w196) -> ("Talon SRX Status"=w195:T11, "CAN Talon SRX Ref"=w197:T5)  [unwired: 8 in, 1 out]
          n82 = Unbundle By Name(w195) -> ("Analog In"=w188:dbl, "Sensor Velocity"=w185:dbl, "Sensor Position"=w194:dbl)
          n83 = Divide(x=w194, y=w186) -> (x/y=w183:dbl)
          n84 = Divide(x=w185, y=w184) -> (x/y=w187:dbl)
          n85 = local write "Actual Position (Rotations) 2"(w183) -> ()
          n86 = Bundle(w183, "Target Value 2"=w189) -> (→"Potentiometer Position Feedback 2":cluster{dbl, "Target Value 2":dbl})  [unwired: 1 in]
          n87 = local write "Actual Speed (RPM) 2"(w187) -> ()
          n88 = local write "A/D Value 2"(w188) -> ()
          n89 = local read "Stop Motor 2"() -> (w181:bool)
          n90 = local read "Stop All"() -> (w180:bool)
          n91 = Or(x=w181, y=w180) -> (x .or. y?=w179:bool)
          n92 = local write "Test Running 2"("Potentiometer Position Control") -> ()
        }
        n93 = call <vilib>:"WPI_MotorControlClose.vi"("MotorControlDevRef"=w178) -> ("error out"=w163:errorcluster)  [unwired: 10 in]
      }
    }
    n94 = local read "Stop All"() -> (w4:bool)
  }
  n95 = while {
    tunnel: "Error In" -> [w202]
    tunnel: [w201] -> w3
    tunnel: [w199] -> w1
    stop <- w199 stop-if-true
    w211 = 360
    n96 = while {
      tunnel: ["P"] -> w210
      tunnel: ["I"] -> w209
      tunnel: ["D"] -> w208
      tunnel: ["F"] -> w207
      tunnel: ["Target Value"] -> w206
      tunnel: ["Control Mode"] -> w205
      tunnel: ["Motor Address"] -> w204
      tunnel: [w219] -> w203
      tunnel: w202 -> [w219]
      tunnel: ["I Zone"] -> w200
      stop <- w215 stop-if-true
      n97 = local read "Start All"() -> (w217:bool)
      n98 = local write "Test Running"("Enter values and press start.") -> ()
      n99 = Or(x=w217, y="Start Motor 1") -> (x .or. y?=w215:bool)
    }
    n100 = Divide(x=w211, y=600) -> (x/y=w212:dbl)
    n101 = case shown="\"Talon Encoder Position\"" w205 {
      tunnel: w212 -> [w236 w271 w328 w357]
      tunnel: w211 -> [w237 w272 w329 _]
      tunnel: w203 -> [w235 w279 w326 _]
      tunnel: [w229 w273 w324 w358] -> w201
      tunnel: w210 -> [w234 w278 _ w362]
      tunnel: w209 -> [w233 w277 _ w361]
      tunnel: w208 -> [w232 w276 _ w356]
      tunnel: w207 -> [w231 w275 _ w360]
      tunnel: w206 -> [w230 w274 w325 w359]
      tunnel: w204 -> [w227 w280 w327 w363]
      tunnel: w200 -> [_ _ _ w355]
      frame "Talon Speed Encoder", Default {
        # "Actual Position (Rotations) = Sensor Position / Encoder Codes Per Rev"
        # "Close reference"
        n102 = call-poly <vilib>:"WPI_MotorControlOpen.vi"("error in (no error)"=w235, "Device Number"=w227, "Control Mode"=WPI_CANTalonSRX_APIControlMode."Speed") -> ("error out"=w241:errorcluster, "MotorControlDeviceRef"=w244:T5)  [unwired: 2 in, 5 out]
        n103 = call <vilib>:"WPI_CANTalonSRX_SetReference.vi"("error in (no error)"=w241, "Reverse Feedback Sensor"=FALSE, "Feedback Reference"=WPI_CANTalonSRX_APIFeedbackSelect."Digital Quadrature Encoder", "CAN Talon SRX Ref"=w244) -> ("error out"=w240:errorcluster, "CAN Talon SRX Ref"=w243:T5)  [unwired: 6 in]
        n104 = call <vilib>:"WPI_CANTalonSRX_SetPID.vi"("CAN Talon SRX Ref"=w243, "P"=w234, "I"=w233, "D"=w232, "error in (no error)"=w240, "F"=w231) -> ("CAN Talon SRX Ref"=w242:T5, "error out"=w239:errorcluster)  [unwired: 8 in]
        n105 = while {
          tunnel: w242 -> [w264]
          tunnel: [w269] -> w247
          tunnel: w236 -> [w263]
          tunnel: w237 -> [w257]
          tunnel: w239 -> [w255]
          tunnel: [w253] -> w238
          tunnel: w230 -> [w252]
          stop <- w248 stop-if-true
          # "loop delay"
          n106 = Multiply(x=w263, y=w252) -> (x*y=w266:dbl)
          n107 = call <vilib>:"WPI_MotorControlSetOutput.vi"("error in (no error)"=w255, "Output"=w266, "MotorControlDevRef"=w264) -> ("error out"=w254:errorcluster, "MotorControlDevRef"=w268:T5)  [unwired: 6 in, 1 out]
          n108 = call <vilib>:"WPI_CANTalonSRX_GetStatus.vi"("error in (no error)"=w254, "CAN Talon SRX Ref"=w268) -> ("error out"=w253:errorcluster, "Talon SRX Status"=w259:T11, "CAN Talon SRX Ref"=w269:T5)  [unwired: 7 in]
          n109 = Wait (ms)(milliseconds to wait=u32 10) -> ()  [unwired: 1 out]
          n110 = Unbundle By Name(w259) -> ("Sensor Velocity"=w267:dbl)
          n111 = Unbundle By Name(w259) -> ("Applied Throttle"=w258:dbl, "Sensor Position"=w256:dbl)
          n112 = Divide(x=w267, y=w263) -> (x/y=w262:dbl)
          n113 = local read "Stop All"() -> (w249:bool)
          n114 = local read "Stop Motor 1"() -> (w250:bool)
          n115 = Bundle(w262, "Target Value"=w252) -> (→"Speed Feedback Chart":cluster{dbl, "Target Value":dbl})  [unwired: 1 in]
          n116 = local write "Actual Speed (RPM)"(w262) -> ()
          n117 = local write "Percent VBus"(w258) -> ()
          n118 = Or(x=w249, y=w250) -> (x .or. y?=w248:bool)
          n119 = Divide(x=w256, y=w257) -> (x/y=w261:dbl)
          n120 = local write "A/D Value"(0) -> ()
          n121 = local write "Actual Position (Rotations)"(w261) -> ()
          n122 = local write "Test Running"("Talon Speed Encoder") -> ()
        }
        n123 = call <vilib>:"WPI_MotorControlClose.vi"("error in (no error)"=w238, "MotorControlDevRef"=w247) -> ("error out"=w229:errorcluster)  [unwired: 9 in]
      }
      frame "Talon Encoder Position" {
        # "Actual Position (Rotations) = Sensor Position / Encoder Codes Per Rev"
        # "Close reference"
        n124 = call-poly <vilib>:"WPI_MotorControlOpen.vi"("error in (no error)"=w279, "Device Number"=w280, "Control Mode"=WPI_CANTalonSRX_APIControlMode."Position") -> ("error out"=w288:errorcluster, "MotorControlDeviceRef"=w285:T5)  [unwired: 2 in, 5 out]
        n125 = call <vilib>:"WPI_CANTalonSRX_SetReference.vi"("error in (no error)"=w288, "Reverse Feedback Sensor"=FALSE, "Feedback Reference"=WPI_CANTalonSRX_APIFeedbackSelect."Digital Quadrature Encoder", "CAN Talon SRX Ref"=w285) -> ("error out"=w289:errorcluster, "CAN Talon SRX Ref"=w286:T5)  [unwired: 6 in]
        n126 = call <vilib>:"WPI_CANTalonSRX_SetPID.vi"("CAN Talon SRX Ref"=w286, "P"=w278, "I"=w277, "D"=w276, "error in (no error)"=w289, "F"=w275) -> ("CAN Talon SRX Ref"=w287:T5, "error out"=w290:errorcluster)  [unwired: 8 in]
        n127 = while {
          tunnel: w287 -> [w308]
          tunnel: [w313] -> w281
          tunnel: w272 -> [w307]
          tunnel: w290 -> [w301]
          tunnel: [w299] -> w291
          tunnel: w274 -> [w298]
          tunnel: w271 -> [w297]
          stop <- w292 stop-if-true
          # "loop delay"
          n128 = Multiply(x=w307, y=w298) -> (x*y=w310:dbl)
          n129 = call <vilib>:"WPI_MotorControlSetOutput.vi"("error in (no error)"=w301, "Output"=w310, "MotorControlDevRef"=w308) -> ("error out"=w300:errorcluster, "MotorControlDevRef"=w312:T5)  [unwired: 6 in, 1 out]
          n130 = call <vilib>:"WPI_CANTalonSRX_GetStatus.vi"("error in (no error)"=w300, "CAN Talon SRX Ref"=w312) -> ("error out"=w299:errorcluster, "Talon SRX Status"=w303:T11, "CAN Talon SRX Ref"=w313:T5)  [unwired: 7 in]
          n131 = Wait (ms)(milliseconds to wait=u32 10) -> ()  [unwired: 1 out]
          n132 = Unbundle By Name(w303) -> ("Sensor Position"=w311:dbl)
          n133 = Unbundle By Name(w303) -> ("Applied Throttle"=w296:dbl, "Sensor Velocity"=w302:dbl)
          n134 = local read "Stop All"() -> (w294:bool)
          n135 = local read "Stop Motor 1"() -> (w293:bool)
          n136 = Divide(x=w311, y=w307) -> (x/y=w306:dbl)
          n137 = local write "Actual Position (Rotations)"(w306) -> ()
          n138 = Bundle(w306, "Target Value"=w298) -> (→"Position Feedback Chart":cluster{dbl, "Target Value":dbl})  [unwired: 1 in]
          n139 = Or(x=w294, y=w293) -> (x .or. y?=w292:bool)
          n140 = local write "Percent VBus"(w296) -> ()
          n141 = Divide(x=w302, y=w297) -> (x/y=w305:dbl)
          n142 = local write "Actual Speed (RPM)"(w305) -> ()
          n143 = local write "A/D Value"(0) -> ()
          n144 = local write "Test Running"("Talon Encoder Position") -> ()
        }
        n145 = call <vilib>:"WPI_MotorControlClose.vi"("error in (no error)"=w291, "MotorControlDevRef"=w281) -> ("error out"=w273:errorcluster)  [unwired: 9 in]
      }
      frame "Voltage Control" {
        # "Close reference"
        n146 = call-poly <vilib>:"WPI_MotorControlOpen.vi"("error in (no error)"=w326, "Device Number"=w327, "Control Mode"=WPI_CANTalonSRX_APIControlMode."Percent VBus") -> ("error out"=w320:errorcluster, "MotorControlDeviceRef"=w323:T5)  [unwired: 2 in, 5 out]
        n147 = call <vilib>:"WPI_CANTalonSRX_ConfigEnabledLimits.vi"("CAN Talon SRX Ref"=w323, "Forward Limit Switch Enable"="Forward Limit Switch", "Reverse Limit Switch Enable"="Reverse Limit Switch", "error in (no error)"=w320) -> ("CAN Talon SRX Ref"=w322:T5, "error out"=w319:errorcluster)  [unwired: 10 in]
        n148 = call <vilib>:"WPI_CANTalonSRX_ConfigLimitSwitches.vi"("CAN Talon SRX Ref"=w322, "Forward Limit Switch Normally Open"="Switches Normally Open", "Reverse Limit Switch Normally Open"="Switches Normally Open", "error in (no error)"=w319) -> ("CAN Talon SRX Ref"=w321:T5, "error out"=w318:errorcluster)  [unwired: 10 in]
        n149 = while {
          tunnel: w321 -> [w350]
          tunnel: [w353] -> w331
          tunnel: w328 -> [w349]
          tunnel: w329 -> [w345]
          tunnel: w318 -> [w341]
          tunnel: [w339] -> w330
          tunnel: w325 -> [w337]
          stop <- w333 stop-if-true
          # "loop delay"
          n150 = Wait (ms)(milliseconds to wait=u32 10) -> ()  [unwired: 1 out]
          n151 = call <vilib>:"WPI_MotorControlSetOutput.vi"("error in (no error)"=w341, "Output"=w337, "MotorControlDevRef"=w350) -> ("error out"=w340:errorcluster, "MotorControlDevRef"=w352:T5)  [unwired: 6 in, 1 out]
          n152 = call <vilib>:"WPI_CANTalonSRX_GetStatus.vi"("error in (no error)"=w340, "CAN Talon SRX Ref"=w352) -> ("error out"=w339:errorcluster, "Talon SRX Status"=w351:T11, "CAN Talon SRX Ref"=w353:T5)  [unwired: 7 in]
          n153 = Unbundle By Name(w351) -> ("Applied Throttle"=w348:dbl, "Sensor Velocity"=w346:dbl, "Sensor Position"=w344:dbl)
          n154 = local read "Stop Motor 1"() -> (w335:bool)
          n155 = local read "Stop All"() -> (w334:bool)
          n156 = Bundle("Applied Throttle"=w348, "Target Value"=w337) -> (→"Voltage Feedback Chart":T13)  [unwired: 1 in]
          n157 = Or(x=w335, y=w334) -> (x .or. y?=w333:bool)
          n158 = Divide(x=w346, y=w349) -> (x/y=w347:dbl)
          n159 = Divide(x=w344, y=w345) -> (x/y=w343:dbl)
          n160 = local write "A/D Value"(0) -> ()
          n161 = local write "Actual Speed (RPM)"(w347) -> ()
          n162 = local write "Test Running"("Voltage Control") -> ()
          n163 = local write "Actual Position (Rotations)"(w343) -> ()
        }
        n164 = call <vilib>:"WPI_MotorControlClose.vi"("error in (no error)"=w330, "MotorControlDevRef"=w331) -> ("error out"=w324:errorcluster)  [unwired: 9 in]
      }
      frame "Potentiometer Position Control" {
        # "Assuming 10 turn\nPot and max A/D\nValue of 1023"
        # "Actual Position (Rotations) = Sensor Position / Encoder Codes Per Rev"
        # "Close reference"
        n165 = call-poly <vilib>:"WPI_MotorControlOpen.vi"("Device Number"=w363, "Control Mode"=WPI_CANTalonSRX_APIControlMode."Position") -> ("MotorControlDeviceRef"=w370:T5)  [unwired: 3 in, 6 out]
        n166 = call <vilib>:"WPI_CANTalonSRX_SetReference.vi"("Reverse Feedback Sensor"=FALSE, "Feedback Reference"=WPI_CANTalonSRX_APIFeedbackSelect."Analog Potentiometer", "CAN Talon SRX Ref"=w370) -> ("CAN Talon SRX Ref"=w369:T5)  [unwired: 7 in, 1 out]
        n167 = call <vilib>:"WPI_CANTalonSRX_SetPID.vi"("CAN Talon SRX Ref"=w369, "P"=w362, "I"=w361, "D"=w356, "F"=w360, "I Zone"=w355) -> ("CAN Talon SRX Ref"=w366:T5)  [unwired: 8 in, 1 out]
        n168 = Divide(x=1023, y=10) -> (x/y=w367:dbl)
        n169 = while {
          tunnel: w366 -> [w387]
          tunnel: [w392] -> w373
          tunnel: w367 -> [w381]
          tunnel: w359 -> [w384]
          tunnel: w357 -> [w379]
          stop <- w374 stop-if-true
          # "loop delay"
          n170 = Multiply(x=w381, y=w384) -> (x*y=w386:dbl)
          n171 = Round To Nearest(number=w386) -> (nearest integer value=w385:dbl)
          n172 = Wait (ms)(milliseconds to wait=u32 10) -> ()  [unwired: 1 out]
          n173 = call <vilib>:"WPI_MotorControlSetOutput.vi"("Output"=w385, "MotorControlDevRef"=w387) -> ("MotorControlDevRef"=w391:T5)  [unwired: 7 in, 2 out]
          n174 = call <vilib>:"WPI_CANTalonSRX_GetStatus.vi"("CAN Talon SRX Ref"=w391) -> ("Talon SRX Status"=w390:T11, "CAN Talon SRX Ref"=w392:T5)  [unwired: 8 in, 1 out]
          n175 = Unbundle By Name(w390) -> ("Analog In"=w383:dbl, "Sensor Velocity"=w380:dbl, "Sensor Position"=w389:dbl)
          n176 = Divide(x=w389, y=w381) -> (x/y=w378:dbl)
          n177 = Divide(x=w380, y=w379) -> (x/y=w382:dbl)
          n178 = local write "Actual Position (Rotations)"(w378) -> ()
          n179 = Bundle(w378, "Target Value"=w384) -> (→"Potentiometer Position Feedback":cluster{dbl, "Target Value":dbl})  [unwired: 1 in]
          n180 = local write "Actual Speed (RPM)"(w382) -> ()
          n181 = local write "A/D Value"(w383) -> ()
          n182 = local read "Stop All"() -> (w376:bool)
          n183 = local read "Stop Motor 1"() -> (w375:bool)
          n184 = Or(x=w376, y=w375) -> (x .or. y?=w374:bool)
          n185 = local write "Test Running"("Potentiometer Position Control") -> ()
        }
        n186 = call <vilib>:"WPI_MotorControlClose.vi"("MotorControlDevRef"=w373) -> ("error out"=w358:errorcluster)  [unwired: 10 in]
      }
    }
    n187 = local read "Stop All"() -> (w199:bool)
  }
  "Error Out" <- w3
  n188 = while {
    tunnel: "Error In" -> [w397]
    tunnel: [w396] -> _
    tunnel: [w394] -> _
    stop <- w394 stop-if-true
    w406 = 360
    n189 = while {
      tunnel: ["P 3"] -> w405
      tunnel: ["I 3"] -> w404
      tunnel: ["D 3"] -> w403
      tunnel: ["F 3"] -> w402
      tunnel: ["Target Value 3"] -> w401
      tunnel: ["Control Mode 3"] -> w400
      tunnel: ["Motor Address 3"] -> w399
      tunnel: [w414] -> w398
      tunnel: w397 -> [w414]
      tunnel: ["I Zone 3"] -> w395
      stop <- w410 stop-if-true
      n190 = local read "Start All"() -> (w412:bool)
      n191 = local write "Test Running 3"("Enter values and press start.") -> ()
      n192 = Or(x=w412, y="Start Motor 3") -> (x .or. y?=w410:bool)
    }
    n193 = Divide(x=w406, y=600) -> (x/y=w407:dbl)
    n194 = case shown="\"Potentiometer Position Control\"" w400 {
      tunnel: w407 -> [w431 w466 w523 w552]
      tunnel: w406 -> [w432 w467 w524 _]
      tunnel: w398 -> [w430 w474 w521 _]
      tunnel: [w424 w468 w519 w553] -> w396
      tunnel: w405 -> [w429 w473 _ w557]
      tunnel: w404 -> [w428 w472 _ w556]
      tunnel: w403 -> [w427 w471 _ w551]
      tunnel: w402 -> [w426 w470 _ w555]
      tunnel: w401 -> [w425 w469 w520 w554]
      tunnel: w399 -> [w422 w475 w522 w558]
      tunnel: w395 -> [_ _ _ w550]
      frame "Talon Speed Encoder", Default {
        # "Actual Position (Rotations) = Sensor Position / Encoder Codes Per Rev"
        # "Close reference"
        n195 = call-poly <vilib>:"WPI_MotorControlOpen.vi"("error in (no error)"=w430, "Device Number"=w422, "Control Mode"=WPI_CANTalonSRX_APIControlMode."Speed") -> ("error out"=w436:errorcluster, "MotorControlDeviceRef"=w439:T5)  [unwired: 2 in, 5 out]
        n196 = call <vilib>:"WPI_CANTalonSRX_SetReference.vi"("error in (no error)"=w436, "Reverse Feedback Sensor"=FALSE, "Feedback Reference"=WPI_CANTalonSRX_APIFeedbackSelect."Digital Quadrature Encoder", "CAN Talon SRX Ref"=w439) -> ("error out"=w435:errorcluster, "CAN Talon SRX Ref"=w438:T5)  [unwired: 6 in]
        n197 = call <vilib>:"WPI_CANTalonSRX_SetPID.vi"("CAN Talon SRX Ref"=w438, "P"=w429, "I"=w428, "D"=w427, "error in (no error)"=w435, "F"=w426) -> ("CAN Talon SRX Ref"=w437:T5, "error out"=w434:errorcluster)  [unwired: 8 in]
        n198 = while {
          tunnel: w437 -> [w459]
          tunnel: [w464] -> w442
          tunnel: w431 -> [w458]
          tunnel: w432 -> [w452]
          tunnel: w434 -> [w450]
          tunnel: [w448] -> w433
          tunnel: w425 -> [w447]
          stop <- w443 stop-if-true
          # "loop delay"
          n199 = Multiply(x=w458, y=w447) -> (x*y=w461:dbl)
          n200 = call <vilib>:"WPI_MotorControlSetOutput.vi"("error in (no error)"=w450, "Output"=w461, "MotorControlDevRef"=w459) -> ("error out"=w449:errorcluster, "MotorControlDevRef"=w463:T5)  [unwired: 6 in, 1 out]
          n201 = call <vilib>:"WPI_CANTalonSRX_GetStatus.vi"("error in (no error)"=w449, "CAN Talon SRX Ref"=w463) -> ("error out"=w448:errorcluster, "Talon SRX Status"=w454:T11, "CAN Talon SRX Ref"=w464:T5)  [unwired: 7 in]
          n202 = Wait (ms)(milliseconds to wait=u32 10) -> ()  [unwired: 1 out]
          n203 = Unbundle By Name(w454) -> ("Sensor Velocity"=w462:dbl)
          n204 = Unbundle By Name(w454) -> ("Applied Throttle"=w453:dbl, "Sensor Position"=w451:dbl)
          n205 = local read "Stop Motor 3"() -> (w444:bool)
          n206 = Divide(x=w462, y=w458) -> (x/y=w457:dbl)
          n207 = local read "Stop All"() -> (w445:bool)
          n208 = Bundle(w457, "Target Value 3"=w447) -> (→"Speed Feedback Chart 3":cluster{dbl, "Target Value 3":dbl})  [unwired: 1 in]
          n209 = local write "Actual Speed (RPM) 3"(w457) -> ()
          n210 = local write "Percent VBus 3"(w453) -> ()
          n211 = Or(x=w444, y=w445) -> (x .or. y?=w443:bool)
          n212 = Divide(x=w451, y=w452) -> (x/y=w456:dbl)
          n213 = local write "A/D Value 3"(0) -> ()
          n214 = local write "Actual Position (Rotations) 3"(w456) -> ()
          n215 = local write "Test Running 3"("Talon Speed Encoder") -> ()
        }
        n216 = call <vilib>:"WPI_MotorControlClose.vi"("error in (no error)"=w433, "MotorControlDevRef"=w442) -> ("error out"=w424:errorcluster)  [unwired: 9 in]
      }
      frame "Talon Encoder Position" {
        # "Actual Position (Rotations) = Sensor Position / Encoder Codes Per Rev"
        # "Close reference"
        n217 = call-poly <vilib>:"WPI_MotorControlOpen.vi"("error in (no error)"=w474, "Device Number"=w475, "Control Mode"=WPI_CANTalonSRX_APIControlMode."Position") -> ("error out"=w483:errorcluster, "MotorControlDeviceRef"=w480:T5)  [unwired: 2 in, 5 out]
        n218 = call <vilib>:"WPI_CANTalonSRX_SetReference.vi"("error in (no error)"=w483, "Reverse Feedback Sensor"=FALSE, "Feedback Reference"=WPI_CANTalonSRX_APIFeedbackSelect."Digital Quadrature Encoder", "CAN Talon SRX Ref"=w480) -> ("error out"=w484:errorcluster, "CAN Talon SRX Ref"=w481:T5)  [unwired: 6 in]
        n219 = call <vilib>:"WPI_CANTalonSRX_SetPID.vi"("CAN Talon SRX Ref"=w481, "P"=w473, "I"=w472, "D"=w471, "error in (no error)"=w484, "F"=w470) -> ("CAN Talon SRX Ref"=w482:T5, "error out"=w485:errorcluster)  [unwired: 8 in]
        n220 = while {
          tunnel: w482 -> [w503]
          tunnel: [w508] -> w476
          tunnel: w467 -> [w502]
          tunnel: w485 -> [w496]
          tunnel: [w494] -> w486
          tunnel: w469 -> [w493]
          tunnel: w466 -> [w492]
          stop <- w487 stop-if-true
          # "loop delay"
          n221 = Multiply(x=w502, y=w493) -> (x*y=w505:dbl)
          n222 = call <vilib>:"WPI_MotorControlSetOutput.vi"("error in (no error)"=w496, "Output"=w505, "MotorControlDevRef"=w503) -> ("error out"=w495:errorcluster, "MotorControlDevRef"=w507:T5)  [unwired: 6 in, 1 out]
          n223 = call <vilib>:"WPI_CANTalonSRX_GetStatus.vi"("error in (no error)"=w495, "CAN Talon SRX Ref"=w507) -> ("error out"=w494:errorcluster, "Talon SRX Status"=w498:T11, "CAN Talon SRX Ref"=w508:T5)  [unwired: 7 in]
          n224 = Wait (ms)(milliseconds to wait=u32 10) -> ()  [unwired: 1 out]
          n225 = Unbundle By Name(w498) -> ("Sensor Position"=w506:dbl)
          n226 = Unbundle By Name(w498) -> ("Applied Throttle"=w491:dbl, "Sensor Velocity"=w497:dbl)
          n227 = local read "Stop Motor 3"() -> (w489:bool)
          n228 = Divide(x=w506, y=w502) -> (x/y=w501:dbl)
          n229 = local read "Stop All"() -> (w488:bool)
          n230 = local write "Actual Position (Rotations) 3"(w501) -> ()
          n231 = Bundle(w501, "Target Value 3"=w493) -> (→"Position Feedback Chart 3":cluster{dbl, "Target Value 3":dbl})  [unwired: 1 in]
          n232 = Or(x=w489, y=w488) -> (x .or. y?=w487:bool)
          n233 = local write "Percent VBus 3"(w491) -> ()
          n234 = Divide(x=w497, y=w492) -> (x/y=w500:dbl)
          n235 = local write "Actual Speed (RPM) 3"(w500) -> ()
          n236 = local write "A/D Value 3"(0) -> ()
          n237 = local write "Test Running 3"("Talon Encoder Position") -> ()
        }
        n238 = call <vilib>:"WPI_MotorControlClose.vi"("error in (no error)"=w486, "MotorControlDevRef"=w476) -> ("error out"=w468:errorcluster)  [unwired: 9 in]
      }
      frame "Voltage Control" {
        # "Close reference"
        n239 = call-poly <vilib>:"WPI_MotorControlOpen.vi"("error in (no error)"=w521, "Device Number"=w522, "Control Mode"=WPI_CANTalonSRX_APIControlMode."Percent VBus") -> ("error out"=w515:errorcluster, "MotorControlDeviceRef"=w518:T5)  [unwired: 2 in, 5 out]
        n240 = call <vilib>:"WPI_CANTalonSRX_ConfigEnabledLimits.vi"("CAN Talon SRX Ref"=w518, "Forward Limit Switch Enable"="Forward Limit Switch 3", "Reverse Limit Switch Enable"="Reverse Limit Switch 3", "error in (no error)"=w515) -> ("CAN Talon SRX Ref"=w517:T5, "error out"=w514:errorcluster)  [unwired: 10 in]
        n241 = call <vilib>:"WPI_CANTalonSRX_ConfigLimitSwitches.vi"("CAN Talon SRX Ref"=w517, "Forward Limit Switch Normally Open"="Switches Normally Open 3", "Reverse Limit Switch Normally Open"="Switches Normally Open 3", "error in (no error)"=w514) -> ("CAN Talon SRX Ref"=w516:T5, "error out"=w513:errorcluster)  [unwired: 10 in]
        n242 = while {
          tunnel: w516 -> [w545]
          tunnel: [w548] -> w526
          tunnel: w523 -> [w544]
          tunnel: w524 -> [w540]
          tunnel: w513 -> [w536]
          tunnel: [w534] -> w525
          tunnel: w520 -> [w532]
          stop <- w528 stop-if-true
          # "loop delay"
          n243 = Wait (ms)(milliseconds to wait=u32 10) -> ()  [unwired: 1 out]
          n244 = call <vilib>:"WPI_MotorControlSetOutput.vi"("error in (no error)"=w536, "Output"=w532, "MotorControlDevRef"=w545) -> ("error out"=w535:errorcluster, "MotorControlDevRef"=w547:T5)  [unwired: 6 in, 1 out]
          n245 = call <vilib>:"WPI_CANTalonSRX_GetStatus.vi"("error in (no error)"=w535, "CAN Talon SRX Ref"=w547) -> ("error out"=w534:errorcluster, "Talon SRX Status"=w546:T11, "CAN Talon SRX Ref"=w548:T5)  [unwired: 7 in]
          n246 = Unbundle By Name(w546) -> ("Applied Throttle"=w543:dbl, "Sensor Velocity"=w541:dbl, "Sensor Position"=w539:dbl)
          n247 = local read "Stop Motor 3"() -> (w530:bool)
          n248 = local read "Stop All"() -> (w529:bool)
          n249 = Bundle("Applied Throttle"=w543, "Target Value 3"=w532) -> (→"Voltage Feedback Chart 3":T14)  [unwired: 1 in]
          n250 = Or(x=w530, y=w529) -> (x .or. y?=w528:bool)
          n251 = Divide(x=w541, y=w544) -> (x/y=w542:dbl)
          n252 = Divide(x=w539, y=w540) -> (x/y=w538:dbl)
          n253 = local write "A/D Value 3"(0) -> ()
          n254 = local write "Actual Speed (RPM) 3"(w542) -> ()
          n255 = local write "Test Running 3"("Voltage Control") -> ()
          n256 = local write "Actual Position (Rotations) 3"(w538) -> ()
        }
        n257 = call <vilib>:"WPI_MotorControlClose.vi"("error in (no error)"=w525, "MotorControlDevRef"=w526) -> ("error out"=w519:errorcluster)  [unwired: 9 in]
      }
      frame "Potentiometer Position Control" {
        # "Assuming 10 turn\nPot and max A/D\nValue of 1023"
        # "Actual Position (Rotations) = Sensor Position / Encoder Codes Per Rev"
        # "Close reference"
        n258 = call-poly <vilib>:"WPI_MotorControlOpen.vi"("Device Number"=w558, "Control Mode"=WPI_CANTalonSRX_APIControlMode."Position") -> ("MotorControlDeviceRef"=w565:T5)  [unwired: 3 in, 6 out]
        n259 = call <vilib>:"WPI_CANTalonSRX_SetReference.vi"("Reverse Feedback Sensor"=FALSE, "Feedback Reference"=WPI_CANTalonSRX_APIFeedbackSelect."Analog Potentiometer", "CAN Talon SRX Ref"=w565) -> ("CAN Talon SRX Ref"=w564:T5)  [unwired: 7 in, 1 out]
        n260 = call <vilib>:"WPI_CANTalonSRX_SetPID.vi"("CAN Talon SRX Ref"=w564, "P"=w557, "I"=w556, "D"=w551, "F"=w555, "I Zone"=w550) -> ("CAN Talon SRX Ref"=w561:T5)  [unwired: 8 in, 1 out]
        n261 = Divide(x=1023, y=10) -> (x/y=w562:dbl)
        n262 = while {
          tunnel: w561 -> [w582]
          tunnel: [w587] -> w568
          tunnel: w562 -> [w576]
          tunnel: w554 -> [w579]
          tunnel: w552 -> [w574]
          stop <- w569 stop-if-true
          # "loop delay"
          n263 = Multiply(x=w576, y=w579) -> (x*y=w581:dbl)
          n264 = Round To Nearest(number=w581) -> (nearest integer value=w580:dbl)
          n265 = Wait (ms)(milliseconds to wait=u32 10) -> ()  [unwired: 1 out]
          n266 = call <vilib>:"WPI_MotorControlSetOutput.vi"("Output"=w580, "MotorControlDevRef"=w582) -> ("MotorControlDevRef"=w586:T5)  [unwired: 7 in, 2 out]
          n267 = call <vilib>:"WPI_CANTalonSRX_GetStatus.vi"("CAN Talon SRX Ref"=w586) -> ("Talon SRX Status"=w585:T11, "CAN Talon SRX Ref"=w587:T5)  [unwired: 8 in, 1 out]
          n268 = Unbundle By Name(w585) -> ("Analog In"=w578:dbl, "Sensor Velocity"=w575:dbl, "Sensor Position"=w584:dbl)
          n269 = Divide(x=w584, y=w576) -> (x/y=w573:dbl)
          n270 = Divide(x=w575, y=w574) -> (x/y=w577:dbl)
          n271 = local write "Actual Position (Rotations) 3"(w573) -> ()
          n272 = Bundle(w573, "Target Value 3"=w579) -> (→"Potentiometer Position Feedback 3":cluster{dbl, "Target Value 3":dbl})  [unwired: 1 in]
          n273 = local write "Actual Speed (RPM) 3"(w577) -> ()
          n274 = local write "A/D Value 3"(w578) -> ()
          n275 = local read "Stop Motor 3"() -> (w571:bool)
          n276 = local read "Stop All"() -> (w570:bool)
          n277 = Or(x=w571, y=w570) -> (x .or. y?=w569:bool)
          n278 = local write "Test Running 3"("Potentiometer Position Control") -> ()
        }
        n279 = call <vilib>:"WPI_MotorControlClose.vi"("MotorControlDevRef"=w568) -> ("error out"=w553:errorcluster)  [unwired: 10 in]
      }
    }
    n280 = local read "Stop All"() -> (w394:bool)
  }
  n281 = while {
    tunnel: "Error In" -> [w592]
    tunnel: [w591] -> _
    tunnel: [w589] -> _
    stop <- w589 stop-if-true
    w601 = 360
    n282 = while {
      tunnel: ["P 4"] -> w600
      tunnel: ["I 4"] -> w599
      tunnel: ["D 4"] -> w598
      tunnel: ["F 4"] -> w597
      tunnel: ["Target Value 4"] -> w596
      tunnel: ["Control Mode 4"] -> w595
      tunnel: ["Motor Address 4"] -> w594
      tunnel: [w609] -> w593
      tunnel: w592 -> [w609]
      tunnel: ["I Zone 4"] -> w590
      stop <- w605 stop-if-true
      n283 = local read "Start All"() -> (w607:bool)
      n284 = local write "Test Running 4"("Enter values and press start.") -> ()
      n285 = Or(x=w607, y="Start Motor 4") -> (x .or. y?=w605:bool)
    }
    n286 = Divide(x=w601, y=600) -> (x/y=w602:dbl)
    n287 = case shown="\"Potentiometer Position Control\"" w595 {
      tunnel: w602 -> [w626 w661 w718 w747]
      tunnel: w601 -> [w627 w662 w719 _]
      tunnel: w593 -> [w625 w669 w716 _]
      tunnel: [w619 w663 w714 w748] -> w591
      tunnel: w600 -> [w624 w668 _ w752]
      tunnel: w599 -> [w623 w667 _ w751]
      tunnel: w598 -> [w622 w666 _ w746]
      tunnel: w597 -> [w621 w665 _ w750]
      tunnel: w596 -> [w620 w664 w715 w749]
      tunnel: w594 -> [w617 w670 w717 w753]
      tunnel: w590 -> [_ _ _ w745]
      frame "Talon Speed Encoder", Default {
        # "Actual Position (Rotations) = Sensor Position / Encoder Codes Per Rev"
        # "Close reference"
        n288 = call-poly <vilib>:"WPI_MotorControlOpen.vi"("error in (no error)"=w625, "Device Number"=w617, "Control Mode"=WPI_CANTalonSRX_APIControlMode."Speed") -> ("error out"=w631:errorcluster, "MotorControlDeviceRef"=w634:T5)  [unwired: 2 in, 5 out]
        n289 = call <vilib>:"WPI_CANTalonSRX_SetReference.vi"("error in (no error)"=w631, "Reverse Feedback Sensor"=FALSE, "Feedback Reference"=WPI_CANTalonSRX_APIFeedbackSelect."Digital Quadrature Encoder", "CAN Talon SRX Ref"=w634) -> ("error out"=w630:errorcluster, "CAN Talon SRX Ref"=w633:T5)  [unwired: 6 in]
        n290 = call <vilib>:"WPI_CANTalonSRX_SetPID.vi"("CAN Talon SRX Ref"=w633, "P"=w624, "I"=w623, "D"=w622, "error in (no error)"=w630, "F"=w621) -> ("CAN Talon SRX Ref"=w632:T5, "error out"=w629:errorcluster)  [unwired: 8 in]
        n291 = while {
          tunnel: w632 -> [w654]
          tunnel: [w659] -> w637
          tunnel: w626 -> [w653]
          tunnel: w627 -> [w647]
          tunnel: w629 -> [w645]
          tunnel: [w643] -> w628
          tunnel: w620 -> [w642]
          stop <- w638 stop-if-true
          # "loop delay"
          n292 = Multiply(x=w653, y=w642) -> (x*y=w656:dbl)
          n293 = call <vilib>:"WPI_MotorControlSetOutput.vi"("error in (no error)"=w645, "Output"=w656, "MotorControlDevRef"=w654) -> ("error out"=w644:errorcluster, "MotorControlDevRef"=w658:T5)  [unwired: 6 in, 1 out]
          n294 = call <vilib>:"WPI_CANTalonSRX_GetStatus.vi"("error in (no error)"=w644, "CAN Talon SRX Ref"=w658) -> ("error out"=w643:errorcluster, "Talon SRX Status"=w649:T11, "CAN Talon SRX Ref"=w659:T5)  [unwired: 7 in]
          n295 = Wait (ms)(milliseconds to wait=u32 10) -> ()  [unwired: 1 out]
          n296 = Unbundle By Name(w649) -> ("Sensor Velocity"=w657:dbl)
          n297 = Unbundle By Name(w649) -> ("Applied Throttle"=w648:dbl, "Sensor Position"=w646:dbl)
          n298 = local read "Stop Motor 4"() -> (w639:bool)
          n299 = Divide(x=w657, y=w653) -> (x/y=w652:dbl)
          n300 = local read "Stop All"() -> (w640:bool)
          n301 = Bundle(w652, "Target Value 4"=w642) -> (→"Speed Feedback Chart 4":cluster{dbl, "Target Value 4":dbl})  [unwired: 1 in]
          n302 = local write "Actual Speed (RPM) 4"(w652) -> ()
          n303 = local write "Percent VBus 4"(w648) -> ()
          n304 = Or(x=w639, y=w640) -> (x .or. y?=w638:bool)
          n305 = Divide(x=w646, y=w647) -> (x/y=w651:dbl)
          n306 = local write "A/D Value 4"(0) -> ()
          n307 = local write "Actual Position (Rotations) 4"(w651) -> ()
          n308 = local write "Test Running 4"("Talon Speed Encoder") -> ()
        }
        n309 = call <vilib>:"WPI_MotorControlClose.vi"("error in (no error)"=w628, "MotorControlDevRef"=w637) -> ("error out"=w619:errorcluster)  [unwired: 9 in]
      }
      frame "Talon Encoder Position" {
        # "Actual Position (Rotations) = Sensor Position / Encoder Codes Per Rev"
        # "Close reference"
        n310 = call-poly <vilib>:"WPI_MotorControlOpen.vi"("error in (no error)"=w669, "Device Number"=w670, "Control Mode"=WPI_CANTalonSRX_APIControlMode."Position") -> ("error out"=w678:errorcluster, "MotorControlDeviceRef"=w675:T5)  [unwired: 2 in, 5 out]
        n311 = call <vilib>:"WPI_CANTalonSRX_SetReference.vi"("error in (no error)"=w678, "Reverse Feedback Sensor"=FALSE, "Feedback Reference"=WPI_CANTalonSRX_APIFeedbackSelect."Digital Quadrature Encoder", "CAN Talon SRX Ref"=w675) -> ("error out"=w679:errorcluster, "CAN Talon SRX Ref"=w676:T5)  [unwired: 6 in]
        n312 = call <vilib>:"WPI_CANTalonSRX_SetPID.vi"("CAN Talon SRX Ref"=w676, "P"=w668, "I"=w667, "D"=w666, "error in (no error)"=w679, "F"=w665) -> ("CAN Talon SRX Ref"=w677:T5, "error out"=w680:errorcluster)  [unwired: 8 in]
        n313 = while {
          tunnel: w677 -> [w698]
          tunnel: [w703] -> w671
          tunnel: w662 -> [w697]
          tunnel: w680 -> [w691]
          tunnel: [w689] -> w681
          tunnel: w664 -> [w688]
          tunnel: w661 -> [w687]
          stop <- w682 stop-if-true
          # "loop delay"
          n314 = Multiply(x=w697, y=w688) -> (x*y=w700:dbl)
          n315 = call <vilib>:"WPI_MotorControlSetOutput.vi"("error in (no error)"=w691, "Output"=w700, "MotorControlDevRef"=w698) -> ("error out"=w690:errorcluster, "MotorControlDevRef"=w702:T5)  [unwired: 6 in, 1 out]
          n316 = call <vilib>:"WPI_CANTalonSRX_GetStatus.vi"("error in (no error)"=w690, "CAN Talon SRX Ref"=w702) -> ("error out"=w689:errorcluster, "Talon SRX Status"=w693:T11, "CAN Talon SRX Ref"=w703:T5)  [unwired: 7 in]
          n317 = Wait (ms)(milliseconds to wait=u32 10) -> ()  [unwired: 1 out]
          n318 = Unbundle By Name(w693) -> ("Sensor Position"=w701:dbl)
          n319 = Unbundle By Name(w693) -> ("Applied Throttle"=w686:dbl, "Sensor Velocity"=w692:dbl)
          n320 = local read "Stop Motor 4"() -> (w684:bool)
          n321 = Divide(x=w701, y=w697) -> (x/y=w696:dbl)
          n322 = local read "Stop All"() -> (w683:bool)
          n323 = local write "Actual Position (Rotations) 4"(w696) -> ()
          n324 = Bundle(w696, "Target Value 4"=w688) -> (→"Position Feedback Chart 4":cluster{dbl, "Target Value 4":dbl})  [unwired: 1 in]
          n325 = Or(x=w684, y=w683) -> (x .or. y?=w682:bool)
          n326 = local write "Percent VBus 4"(w686) -> ()
          n327 = Divide(x=w692, y=w687) -> (x/y=w695:dbl)
          n328 = local write "Actual Speed (RPM) 4"(w695) -> ()
          n329 = local write "A/D Value 4"(0) -> ()
          n330 = local write "Test Running 4"("Talon Encoder Position") -> ()
        }
        n331 = call <vilib>:"WPI_MotorControlClose.vi"("error in (no error)"=w681, "MotorControlDevRef"=w671) -> ("error out"=w663:errorcluster)  [unwired: 9 in]
      }
      frame "Voltage Control" {
        # "Close reference"
        n332 = call-poly <vilib>:"WPI_MotorControlOpen.vi"("error in (no error)"=w716, "Device Number"=w717, "Control Mode"=WPI_CANTalonSRX_APIControlMode."Percent VBus") -> ("error out"=w710:errorcluster, "MotorControlDeviceRef"=w713:T5)  [unwired: 2 in, 5 out]
        n333 = call <vilib>:"WPI_CANTalonSRX_ConfigEnabledLimits.vi"("CAN Talon SRX Ref"=w713, "Forward Limit Switch Enable"="Forward Limit Switch 4", "Reverse Limit Switch Enable"="Reverse Limit Switch 4", "error in (no error)"=w710) -> ("CAN Talon SRX Ref"=w712:T5, "error out"=w709:errorcluster)  [unwired: 10 in]
        n334 = call <vilib>:"WPI_CANTalonSRX_ConfigLimitSwitches.vi"("CAN Talon SRX Ref"=w712, "Forward Limit Switch Normally Open"="Switches Normally Open 4", "Reverse Limit Switch Normally Open"="Switches Normally Open 4", "error in (no error)"=w709) -> ("CAN Talon SRX Ref"=w711:T5, "error out"=w708:errorcluster)  [unwired: 10 in]
        n335 = while {
          tunnel: w711 -> [w740]
          tunnel: [w743] -> w721
          tunnel: w718 -> [w739]
          tunnel: w719 -> [w735]
          tunnel: w708 -> [w731]
          tunnel: [w729] -> w720
          tunnel: w715 -> [w727]
          stop <- w723 stop-if-true
          # "loop delay"
          n336 = Wait (ms)(milliseconds to wait=u32 10) -> ()  [unwired: 1 out]
          n337 = call <vilib>:"WPI_MotorControlSetOutput.vi"("error in (no error)"=w731, "Output"=w727, "MotorControlDevRef"=w740) -> ("error out"=w730:errorcluster, "MotorControlDevRef"=w742:T5)  [unwired: 6 in, 1 out]
          n338 = call <vilib>:"WPI_CANTalonSRX_GetStatus.vi"("error in (no error)"=w730, "CAN Talon SRX Ref"=w742) -> ("error out"=w729:errorcluster, "Talon SRX Status"=w741:T11, "CAN Talon SRX Ref"=w743:T5)  [unwired: 7 in]
          n339 = Unbundle By Name(w741) -> ("Applied Throttle"=w738:dbl, "Sensor Velocity"=w736:dbl, "Sensor Position"=w734:dbl)
          n340 = local read "Start Motor 4"() -> (w725:bool)
          n341 = local read "Stop All"() -> (w724:bool)
          n342 = Bundle("Applied Throttle"=w738, "Target Value 4"=w727) -> (→"Voltage Feedback Chart 4":T15)  [unwired: 1 in]
          n343 = Or(x=w725, y=w724) -> (x .or. y?=w723:bool)
          n344 = Divide(x=w736, y=w739) -> (x/y=w737:dbl)
          n345 = Divide(x=w734, y=w735) -> (x/y=w733:dbl)
          n346 = local write "A/D Value 4"(0) -> ()
          n347 = local write "Actual Speed (RPM) 4"(w737) -> ()
          n348 = local write "Test Running 4"("Voltage Control") -> ()
          n349 = local write "Actual Position (Rotations) 4"(w733) -> ()
        }
        n350 = call <vilib>:"WPI_MotorControlClose.vi"("error in (no error)"=w720, "MotorControlDevRef"=w721) -> ("error out"=w714:errorcluster)  [unwired: 9 in]
      }
      frame "Potentiometer Position Control" {
        # "Assuming 10 turn\nPot and max A/D\nValue of 1023"
        # "Actual Position (Rotations) = Sensor Position / Encoder Codes Per Rev"
        # "Close reference"
        n351 = call-poly <vilib>:"WPI_MotorControlOpen.vi"("Device Number"=w753, "Control Mode"=WPI_CANTalonSRX_APIControlMode."Position") -> ("MotorControlDeviceRef"=w760:T5)  [unwired: 3 in, 6 out]
        n352 = call <vilib>:"WPI_CANTalonSRX_SetReference.vi"("Reverse Feedback Sensor"=FALSE, "Feedback Reference"=WPI_CANTalonSRX_APIFeedbackSelect."Analog Potentiometer", "CAN Talon SRX Ref"=w760) -> ("CAN Talon SRX Ref"=w759:T5)  [unwired: 7 in, 1 out]
        n353 = call <vilib>:"WPI_CANTalonSRX_SetPID.vi"("CAN Talon SRX Ref"=w759, "P"=w752, "I"=w751, "D"=w746, "F"=w750, "I Zone"=w745) -> ("CAN Talon SRX Ref"=w756:T5)  [unwired: 8 in, 1 out]
        n354 = Divide(x=1023, y=10) -> (x/y=w757:dbl)
        n355 = while {
          tunnel: w756 -> [w777]
          tunnel: [w782] -> w763
          tunnel: w757 -> [w771]
          tunnel: w749 -> [w774]
          tunnel: w747 -> [w769]
          stop <- w764 stop-if-true
          # "loop delay"
          n356 = Multiply(x=w771, y=w774) -> (x*y=w776:dbl)
          n357 = Round To Nearest(number=w776) -> (nearest integer value=w775:dbl)
          n358 = Wait (ms)(milliseconds to wait=u32 10) -> ()  [unwired: 1 out]
          n359 = call <vilib>:"WPI_MotorControlSetOutput.vi"("Output"=w775, "MotorControlDevRef"=w777) -> ("MotorControlDevRef"=w781:T5)  [unwired: 7 in, 2 out]
          n360 = call <vilib>:"WPI_CANTalonSRX_GetStatus.vi"("CAN Talon SRX Ref"=w781) -> ("Talon SRX Status"=w780:T11, "CAN Talon SRX Ref"=w782:T5)  [unwired: 8 in, 1 out]
          n361 = Unbundle By Name(w780) -> ("Analog In"=w773:dbl, "Sensor Velocity"=w770:dbl, "Sensor Position"=w779:dbl)
          n362 = Divide(x=w779, y=w771) -> (x/y=w768:dbl)
          n363 = Divide(x=w770, y=w769) -> (x/y=w772:dbl)
          n364 = local write "Actual Position (Rotations) 4"(w768) -> ()
          n365 = Bundle(w768, "Target Value 4"=w774) -> (→"Potentiometer Position Feedback 4":cluster{dbl, "Target Value 4":dbl})  [unwired: 1 in]
          n366 = local write "Actual Speed (RPM) 4"(w772) -> ()
          n367 = local write "A/D Value 4"(w773) -> ()
          n368 = local read "Stop Motor 4"() -> (w766:bool)
          n369 = local read "Stop All"() -> (w765:bool)
          n370 = Or(x=w766, y=w765) -> (x .or. y?=w764:bool)
          n371 = local write "Test Running 4"("Potentiometer Position Control") -> ()
        }
        n372 = call <vilib>:"WPI_MotorControlClose.vi"("MotorControlDevRef"=w763) -> ("error out"=w748:errorcluster)  [unwired: 10 in]
      }
    }
    n373 = local read "Stop All"() -> (w589:bool)
  }
  n374 = flat-sequence {
    tunnel: w1 -> [w785]
    tunnel: w3 -> [w784]
    tunnel: [w784] -> _
    frame #0 {
      n375 = Stop(stop? (T)=w785) -> ()
    }
  }
